vi "MPX Panel.vi"(8 "error in":errorcluster, 11 "session in":T1={"niScope"={"channel cfg"=[], "sessions"=[], "multi cards"=FALSE, "channels"=0, "type"=enum."n/a", "memory [B/chn]"=0, "ext. clock [Hz]"=0.0, "samples count"=0, "use streaming"=FALSE, "proc setup"={"packet size [smpl]"=0, "current timeout [s]"=0.0, "blk2blk timeout [s]"=0.0, "event time"=timestamp(0 s since 1904-01-01), "temp sampl T [s]"=0.0, "data queue"=refnum, "stop notifier"=refnum, "proc ref"=refnum}, "sample width [B]"=0, "ranges [V]"=[], "trigger setup"={"coupling"=1, "level [V]"=0.0, "slope"=0, "mode"=enum."Immediate"}, "fs [Hz]"=0.0, "bitres [bit]"=0, "clock source"=enum."VAL_NO_SOURCE"}, "3458A"={"channels"=[], "sync unit"={"VISA"="", "type"=enum."Picotest U6200A"}, "awg unit"={"type"=enum."Agilent 331xxA to 332xxA", "VISA"="", "enable 10MHz ref"=FALSE, "cmi ckd2"={"VISA"="", "clock source"=enum."Auto", "manual ref clk"=FALSE, "ref clock [Hz]"=0.0, "div mode"=enum."Set divisor directly"}, "cmi sync v3"={"VISA"="", "baud rate [bd/s]"=115200, "source"=enum."Auto", "hv range"=enum."1kV", "fsrc is fixed"=FALSE, "fsrc [Hz]"=10000000.0, "freq integ [s]"=1.0, "freq filter"=5, "trig level"=enum."TTL 5V", "chn1 mode"=enum."Source divider", "chn1 level"=enum."Positive 5V", "chn2 mode"=enum."Source divider", "chn2 level"=enum."Positive 5V", "chn2 div"=1, "chn3 mode"=enum."Chn 1 Active", "chn3 level"=enum."Positive 5V", "chn1 div entry"=enum."Calculate nearest divisor from measured fx", "chn1 dev limit [%]"=1.0, "chn1 check dev"=FALSE}, "trigger"={"source"=enum."Immediate", "level [V]"=0.0, "coupling"=enum."DC", "slope"=enum."POS"}, "HMF2500 cfg"={"Baud Rate"=9600, "Parity"=0, "Data Bits"=8, "Flow Control"=4}}, "sync mode"=enum."MASTER-SLAVE, MASTER clocked by TIMER", "streaming mode"=FALSE, "idn mode"=enum."Auto", "sampling mode"=enum."DCV", "sample memory [B]"=0, "proc setup"={"channel id"=0, "packet size [smpl]"=0, "current timeout [s]"=0.0, "blk2blk timeout [s]"=0.0, "event time"=timestamp(0 s since 1904-01-01), "stop notifier"=refnum, "data queues"=[], "proc refs"=[], "bus semaphore"=refnum}, "sample size [B]"=0, "sample count"=0, "aux data"={"channel id"=0, "valid?"=[], "gain [V]"=[], "timestamp [s]"=[], "Ts [s]"=0.0, "abs timestamp"=timestamp(0 s since 1904-01-01), "t [deg C]"=[], "multiplex timestamp [s]"=-1.0, "only multiplex?"=FALSE, "multiplex smpl offset"=0, "overflow?"=FALSE}, "ranges [V]"=[], "aperture [s]"=0.0, "LEVEL trigger"={"edge"=enum."POS", "level [V]"=0.0, "coupling"=enum."DC"}, "trigger mode"=enum."AUTO", "measure temp.?"=FALSE, "disp mesages"=[], "shared bus?"=FALSE, "disable display?"=FALSE, "aper mode"=enum."Manual", "aper rules"=[], "multiplex"={"cycles"=0, "delay [s]"=0.0, "enabled"=FALSE, "overhead [s]"=1.0, "tot smpls"=0, "sub-rec"=0, "overhead [%]"=0.0, "emulated"=FALSE}, "F8588 lpf"=enum."Off", "F8588 pll"=enum."Off", "F8588 couple"=enum."DC, auto", "fs"={"freq mode"=enum."fs or Ts", "fs [Hz]"=0.0, "fref [Hz]"=0.0, "mul"=0.0, "div"=0.0}}, "dsdll"={"dsdll"={"dsdll path"=path "", "dsdll handle"=[], "output devices"=[], "capture devices"=[]}, "channels"=0, "device id"=0, "channel idns"=[], "proc setup"={"packet size [smpl]"=0, "current timeout [s]"=0.0, "blk2blk timeout [s]"=0.0, "event time"=timestamp(0 s since 1904-01-01), "data queue"=refnum, "stop notifier"=refnum, "proc ref"=refnum}, "samples count"=0, "fs [Hz]"=0.0}, "type"=enum."niScope", "channel idn str"=[], "aux instr idn str"=[], "modified?"=FALSE, "simadc"={"channels"=[], "range [V]"=0.0, "Ts step [s]"=0.0, "time [s]"=0.0, "fs [Hz]"=0.0, "count"=0, "smpl offset"=0, "set count"=0, "bit res"=0}, "force rst?"=FALSE, "exit mode"=enum."Immediate reset", "exit dly"=0.0, "exit tmr"=timestamp(0 s since 1904-01-01), "busy?"=FALSE, "accessed?"=FALSE, "multiplex"={"Type"=enum."Dummy", "gen com ssn"={"visa"="", "primary"=enum."None", "secondary"=enum."None", "channels"=[]}, "delay before [s]"=0.0, "delay post [s]"=0.0, "sequence"=[], "enabled"=FALSE, "ref timestamp [s]"=0.0, "idn string"="", "dev niScope"="", "niScope idx"=0, "QPMX ssn"={"visa"="", "switch mode"=enum."Switched by TWM", "sequence"=[], "timing delays"=[], "polarity"=enum."Positive", "ss delay (s)"=2.0, "internal timer (s)"=1.0, "Last loaded sequence file"=path ""}, "VISA mux ssn"={"VISA"="", "paths"=[], "idn command"="", "serial cfg"={"Baud rate"=9600, "Data bits"=8, "Parity"=0, "Stop bits"=10, "Flow control"=0, "End Mode Read"=enum."None", "End Mode Write"=enum."None", "Term character"=0, "Term enable"=FALSE}}}, "keysight dso"={"VISA"="", "channels"=[], "bw limit [Hz]"=0.0, "resolution"=enum."Auto", "trig noise reject"=enum."Normal", "N"=0, "trigger config"={"trigger source"=enum."Immediate", "level [V]"=0.0, "trigger slope"=enum."Negative"}, "fs [Hz]"=0.0, "timeout stop"=timestamp(0 s since 1904-01-01), "waiting for opc"=FALSE, "fetch offset [smpl]"=0, "abs timestamp"=timestamp(0 s since 1904-01-01), "ranges [V]"=[]}, "cdaq"={"mclk [Hz]"=12800000.0, "ADC task"="", "mclk reference"="", "fs [Hz]"=50000.0, "queue adc cmd"=refnum, "queue adc data"=refnum, "adc proc ref"=refnum, "channels"=[], "last channels"=[], "timeout"=timestamp(0 s since 1904-01-01), "N"=1000, "mclk mode"=enum."Free running", "ext mclk source"=""}, "ignore overload"=FALSE} {"cdaq"."last channels"."Channel id" min=0 step=1; "cdaq"."channels"."Channel id" min=0 step=1; "keysight dso"."bw limit [Hz]" format="%#_6p"; "keysight dso"."channels"."Offset [V]" min=0.0 format="%#_6p"; "keysight dso"."channels"."Range [Vpk]" min=0.0 format="%#_6p"; "keysight dso"."channels"."Channel" min=1; "multiplex"."VISA mux ssn"."serial cfg"."Flow control" items=["None", "XON/XOFF", "CTS/RTS", "XON/XOFF + CTS/RTS", "DTR/DSR", "XON/XOFF + DTR/DSR"]; "multiplex"."VISA mux ssn"."serial cfg"."Stop bits" items=["1 bit"=10, "1.5 bits"=15, "2 bits"=20]; "multiplex"."VISA mux ssn"."serial cfg"."Parity" items=["None", "Odd", "Even", "Mark", "Space"]; "multiplex"."VISA mux ssn"."serial cfg"."Data bits" items=["5 bits"=5, "6 bits"=6, "7 bits"=7, "8 bits"=8]; "multiplex"."VISA mux ssn"."serial cfg"."Baud rate" items=["150 Bd"=150, "300 Bd"=300, "600 Bd"=600, "1200 Bd"=1200, "2400 Bd"=2400, "4800 Bd"=4800, "9600 Bd"=9600, "19.2 kBd"=19200, "38.4 kBd"=38400, "57.6 kBd"=57600, "115.2 kBd"=115200]; "multiplex"."QPMX ssn"."internal timer (s)" min=0.0 step=1.0; "multiplex"."QPMX ssn"."ss delay (s)" min=0.0 step=1.0; "multiplex"."QPMX ssn"."timing delays" min=1 max=255 step=1; "3458A"."awg unit"."HMF2500 cfg"."Flow Control" items=["None", "XON/XOFF", "RTS/CTS", "XON/XOFF & RTS/CTS", "DTR/DSR", "XON/XOFF & DTR/DSR"]; "3458A"."awg unit"."HMF2500 cfg"."Data Bits" items=["7"=7, "8"=8]; "3458A"."awg unit"."HMF2500 cfg"."Parity" items=["None", "Odd", "Even", "Mark", "Space"]; "3458A"."awg unit"."HMF2500 cfg"."Baud Rate" items=["300"=300, "600"=600, "1200"=1200, "2400"=2400, "4800"=4800, "9600"=9600, "19200"=19200]; "3458A"."awg unit"."cmi sync v3"."chn2 div" min=1 max=100000000 step=1; "3458A"."awg unit"."cmi sync v3"."fsrc [Hz]" format="%_8p"; "3458A"."channels"."Range [Vpk]" min=0.0; "niScope"."trigger setup"."level [V]" format="%.2f"; "niScope"."trigger setup"."coupling" items=["AC"=0, "DC"=1, "HF Reject"=3, "LF Reject"=4, "AC Plus HF Reject"=1001]; "niScope"."channel cfg"."Range [Vpk]" min=0.0; "niScope"."channel cfg"."Channel" min=0}) -> (0 "error out":errorcluster, 3 "session out":T1={"niScope"={"channel cfg"=[], "sessions"=[], "multi cards"=FALSE, "channels"=0, "type"=enum."n/a", "memory [B/chn]"=0, "ext. clock [Hz]"=0.0, "samples count"=0, "use streaming"=FALSE, "proc setup"={"packet size [smpl]"=0, "current timeout [s]"=0.0, "blk2blk timeout [s]"=0.0, "event time"=timestamp(0 s since 1904-01-01), "temp sampl T [s]"=0.0, "data queue"=refnum, "stop notifier"=refnum, "proc ref"=refnum}, "sample width [B]"=0, "ranges [V]"=[], "trigger setup"={"coupling"=1, "level [V]"=0.0, "slope"=0, "mode"=enum."Immediate"}, "fs [Hz]"=0.0, "bitres [bit]"=0, "clock source"=enum."VAL_NO_SOURCE"}, "3458A"={"channels"=[], "sync unit"={"VISA"="", "type"=enum."Picotest U6200A"}, "awg unit"={"type"=enum."Agilent 331xxA to 332xxA", "VISA"="", "enable 10MHz ref"=FALSE, "cmi ckd2"={"VISA"="", "clock source"=enum."Auto", "manual ref clk"=FALSE, "ref clock [Hz]"=0.0, "div mode"=enum."Set divisor directly"}, "cmi sync v3"={"VISA"="", "baud rate [bd/s]"=115200, "source"=enum."Auto", "hv range"=enum."1kV", "fsrc is fixed"=FALSE, "fsrc [Hz]"=10000000.0, "freq integ [s]"=1.0, "freq filter"=5, "trig level"=enum."TTL 5V", "chn1 mode"=enum."Source divider", "chn1 level"=enum."Positive 5V", "chn2 mode"=enum."Source divider", "chn2 level"=enum."Positive 5V", "chn2 div"=1, "chn3 mode"=enum."Chn 1 Active", "chn3 level"=enum."Positive 5V", "chn1 div entry"=enum."Calculate nearest divisor from measured fx", "chn1 dev limit [%]"=1.0, "chn1 check dev"=FALSE}, "trigger"={"source"=enum."Immediate", "level [V]"=0.0, "coupling"=enum."DC", "slope"=enum."POS"}, "HMF2500 cfg"={"Baud Rate"=9600, "Parity"=0, "Data Bits"=8, "Flow Control"=4}}, "sync mode"=enum."MASTER-SLAVE, MASTER clocked by TIMER", "streaming mode"=FALSE, "idn mode"=enum."Auto", "sampling mode"=enum."DCV", "sample memory [B]"=0, "proc setup"={"channel id"=0, "packet size [smpl]"=0, "current timeout [s]"=0.0, "blk2blk timeout [s]"=0.0, "event time"=timestamp(0 s since 1904-01-01), "stop notifier"=refnum, "data queues"=[], "proc refs"=[], "bus semaphore"=refnum}, "sample size [B]"=0, "sample count"=0, "aux data"={"channel id"=0, "valid?"=[], "gain [V]"=[], "timestamp [s]"=[], "Ts [s]"=0.0, "abs timestamp"=timestamp(0 s since 1904-01-01), "t [deg C]"=[], "multiplex timestamp [s]"=-1.0, "only multiplex?"=FALSE, "multiplex smpl offset"=0, "overflow?"=FALSE}, "ranges [V]"=[], "aperture [s]"=0.0, "LEVEL trigger"={"edge"=enum."POS", "level [V]"=0.0, "coupling"=enum."DC"}, "trigger mode"=enum."AUTO", "measure temp.?"=FALSE, "disp mesages"=[], "shared bus?"=FALSE, "disable display?"=FALSE, "aper mode"=enum."Manual", "aper rules"=[], "multiplex"={"cycles"=0, "delay [s]"=0.0, "enabled"=FALSE, "overhead [s]"=1.0, "tot smpls"=0, "sub-rec"=0, "overhead [%]"=0.0, "emulated"=FALSE}, "F8588 lpf"=enum."Off", "F8588 pll"=enum."Off", "F8588 couple"=enum."DC, auto", "fs"={"freq mode"=enum."fs or Ts", "fs [Hz]"=0.0, "fref [Hz]"=0.0, "mul"=0.0, "div"=0.0}}, "dsdll"={"dsdll"={"dsdll path"=path "", "dsdll handle"=[], "output devices"=[], "capture devices"=[]}, "channels"=0, "device id"=0, "channel idns"=[], "proc setup"={"packet size [smpl]"=0, "current timeout [s]"=0.0, "blk2blk timeout [s]"=0.0, "event time"=timestamp(0 s since 1904-01-01), "data queue"=refnum, "stop notifier"=refnum, "proc ref"=refnum}, "samples count"=0, "fs [Hz]"=0.0}, "type"=enum."niScope", "channel idn str"=[], "aux instr idn str"=[], "modified?"=FALSE, "simadc"={"channels"=[], "range [V]"=0.0, "Ts step [s]"=0.0, "time [s]"=0.0, "fs [Hz]"=0.0, "count"=0, "smpl offset"=0, "set count"=0, "bit res"=0}, "force rst?"=FALSE, "exit mode"=enum."Immediate reset", "exit dly"=0.0, "exit tmr"=timestamp(0 s since 1904-01-01), "busy?"=FALSE, "accessed?"=FALSE, "multiplex"={"Type"=enum."Dummy", "gen com ssn"={"visa"="", "primary"=enum."None", "secondary"=enum."None", "channels"=[]}, "delay before [s]"=0.0, "delay post [s]"=0.0, "sequence"=[], "enabled"=FALSE, "ref timestamp [s]"=0.0, "idn string"="", "dev niScope"="", "niScope idx"=0, "QPMX ssn"={"visa"="", "switch mode"=enum."Switched by TWM", "sequence"=[], "timing delays"=[], "polarity"=enum."Positive", "ss delay (s)"=2.0, "internal timer (s)"=1.0, "Last loaded sequence file"=path ""}, "VISA mux ssn"={"VISA"="", "paths"=[], "idn command"="", "serial cfg"={"Baud rate"=9600, "Data bits"=8, "Parity"=0, "Stop bits"=10, "Flow control"=0, "End Mode Read"=enum."None", "End Mode Write"=enum."None", "Term character"=0, "Term enable"=FALSE}}}, "keysight dso"={"VISA"="", "channels"=[], "bw limit [Hz]"=0.0, "resolution"=enum."Auto", "trig noise reject"=enum."Normal", "N"=0, "trigger config"={"trigger source"=enum."Immediate", "level [V]"=0.0, "trigger slope"=enum."Negative"}, "fs [Hz]"=0.0, "timeout stop"=timestamp(0 s since 1904-01-01), "waiting for opc"=FALSE, "fetch offset [smpl]"=0, "abs timestamp"=timestamp(0 s since 1904-01-01), "ranges [V]"=[]}, "cdaq"={"mclk [Hz]"=12800000.0, "ADC task"="", "mclk reference"="", "fs [Hz]"=50000.0, "queue adc cmd"=refnum, "queue adc data"=refnum, "adc proc ref"=refnum, "channels"=[], "last channels"=[], "timeout"=timestamp(0 s since 1904-01-01), "N"=1000, "mclk mode"=enum."Free running", "ext mclk source"=""}, "ignore overload"=FALSE} {"cdaq"."last channels"."Channel id" min=0 step=1; "cdaq"."channels"."Channel id" min=0 step=1; "keysight dso"."bw limit [Hz]" format="%#_6p"; "keysight dso"."channels"."Offset [V]" min=0.0 format="%#_6p"; "keysight dso"."channels"."Range [Vpk]" min=0.0 format="%#_6p"; "keysight dso"."channels"."Channel" min=1; "multiplex"."VISA mux ssn"."serial cfg"."Flow control" items=["None", "XON/XOFF", "CTS/RTS", "XON/XOFF + CTS/RTS", "DTR/DSR", "XON/XOFF + DTR/DSR"]; "multiplex"."VISA mux ssn"."serial cfg"."Stop bits" items=["1 bit"=10, "1.5 bits"=15, "2 bits"=20]; "multiplex"."VISA mux ssn"."serial cfg"."Parity" items=["None", "Odd", "Even", "Mark", "Space"]; "multiplex"."VISA mux ssn"."serial cfg"."Data bits" items=["5 bits"=5, "6 bits"=6, "7 bits"=7, "8 bits"=8]; "multiplex"."VISA mux ssn"."serial cfg"."Baud rate" items=["150 Bd"=150, "300 Bd"=300, "600 Bd"=600, "1200 Bd"=1200, "2400 Bd"=2400, "4800 Bd"=4800, "9600 Bd"=9600, "19.2 kBd"=19200, "38.4 kBd"=38400, "57.6 kBd"=57600, "115.2 kBd"=115200]; "multiplex"."QPMX ssn"."internal timer (s)" min=0.0 step=1.0; "multiplex"."QPMX ssn"."ss delay (s)" min=0.0 step=1.0; "multiplex"."QPMX ssn"."timing delays" min=1 max=255 step=1; "3458A"."awg unit"."HMF2500 cfg"."Flow Control" items=["None", "XON/XOFF", "RTS/CTS", "XON/XOFF & RTS/CTS", "DTR/DSR", "XON/XOFF & DTR/DSR"]; "3458A"."awg unit"."HMF2500 cfg"."Data Bits" items=["7"=7, "8"=8]; "3458A"."awg unit"."HMF2500 cfg"."Parity" items=["None", "Odd", "Even", "Mark", "Space"]; "3458A"."awg unit"."HMF2500 cfg"."Baud Rate" items=["300"=300, "600"=600, "1200"=1200, "2400"=2400, "4800"=4800, "9600"=9600, "19200"=19200]; "3458A"."awg unit"."cmi sync v3"."chn2 div" min=1 max=100000000 step=1; "3458A"."awg unit"."cmi sync v3"."fsrc [Hz]" format="%_8p"; "3458A"."channels"."Range [Vpk]" min=0.0; "niScope"."trigger setup"."level [V]" format="%.2f"; "niScope"."trigger setup"."coupling" items=["AC"=0, "DC"=1, "HF Reject"=3, "LF Reject"=4, "AC Plus HF Reject"=1001]; "niScope"."channel cfg"."Range [Vpk]" min=0.0; "niScope"."channel cfg"."Channel" min=0})   [LabVIEW 2020]
doc: "Multiplexer configuration panel."
uses:
  drivers/Multiplexers/Generic VISA commands/GVISA Mux Path Entry.ctl
  MPX Type.ctl
  drivers/Multiplexers/Generic COM/GCOMM Signal.ctl
  drivers/Multiplexers/Generic COM/GCOMM Virtual Channel.ctl
  drivers/Multiplexers/Generic COM/GCOMM Logic State.ctl
  ADC Session.ctl
  drivers/niScope/niScope Session.ctl
  drivers/niScope/niScope Virtual Channel Config.ctl
  drivers/niScope/niScope Virtual Channel Mode.ctl
  drivers/niScope/niScope Virtual Channel Input Z.ctl
  drivers/niScope/niScope Virtual Channel Coupling.ctl
  drivers/niScope/niScope Type.ctl
  drivers/niScope/niScope Digitizing Process Options.ctl
  drivers/niScope/niScope Data Packet.ctl
  drivers/niScope/niScope Trigger Setup.ctl
  <instrlib>/niScope/Controls/niScope trigger coupling.ctl
  <instrlib>/niScope/Controls/niScope trigger slope.ctl
  drivers/niScope/niScope Reference Clock.ctl
  drivers/DMM/3458A Digitizer Session.ctl
  drivers/DMM/3458A Virtual Channel Config.ctl
  drivers/Counter/Counter Session.ctl
  drivers/Counter/Counter Type.ctl
  drivers/AWG/AWG Session.ctl
  drivers/AWG/AWG Type.ctl
  drivers/AWG/CMI Clock Divider v2/CMI ckd2 Session.ctl
  drivers/AWG/CMI Clock Divider v2/CMI ckd2 Source Mode.ctl
  drivers/AWG/CMI Clock Divider v2/CMI ckd2 Divisor Mode.ctl
  drivers/AWG/CMI Sync V3/CMI Sync V3 session.ctl
  drivers/AWG/CMI Sync V3/Configure/CMI Sync V3 Reference Clock Source.ctl
  drivers/AWG/CMI Sync V3/Configure/CMI Sync V3 HV input Range.ctl
  drivers/AWG/CMI Sync V3/Configure/CMI Sync V3 Trigger Input Level.ctl
  drivers/AWG/CMI Sync V3/Configure/CMI Sync V3 Channel 1 Mode.ctl
  drivers/AWG/CMI Sync V3/Configure/CMI Sync V3 Channel Output Levels.ctl
  drivers/AWG/CMI Sync V3/Configure/CMI Sync V3 Channel 2 Mode.ctl
  drivers/AWG/CMI Sync V3/Configure/CMI Sync V3 Channel 3 Mode.ctl
  drivers/AWG/CMI Sync V3/Configure/CMI Sync V3 Channel 1 Divisor Entry Mode.ctl
  ADC Trig Config.ctl
  ADC Trig Mode Source.ctl
  ADC Trig Coupling.ctl
  ADC Trig Slope.ctl
  drivers/AWG/RaS HMF2500/HMF2500 Config.ctl
  drivers/DMM/3458A Sync Mode.ctl
  drivers/DMM/3458A Idn Mode.ctl
  drivers/DMM/3458A Digitizing Low Levels/Configure/Sampling Mode.ctl
  drivers/DMM/3458A Digitizing Process Options.ctl
  drivers/DMM/3458A Data Packet.ctl
  drivers/DMM/3458A Aux Record Data.ctl
  drivers/DMM/3458A Digitizing Low Levels/Configure/Level Setup.ctl
  drivers/DMM/3458A Digitizing Low Levels/Configure/First Sample Trigger.ctl
  drivers/DMM/3458A Aperture Selection Mode.ctl
  drivers/DMM/3458A Multiplexing Config.ctl
  drivers/Fluke 8588A/F8588A Low Pass Filter.ctl
  drivers/Fluke 8588A/F8588A Phase Lock.ctl
  drivers/Fluke 8588A/F8588A Coupling.ctl
  drivers/DMM/3458A Sampling Rate.ctl
  drivers/AWG/AWG Clock Setup Mode.ctl
  drivers/dsdll/DSDLL Session.ctl
  drivers/dsdll/dsdll/dsdll_instance.ctl
  drivers/dsdll/dsdll/dsdll_device_record.ctl
  drivers/dsdll/DSDLL Process Config.ctl
  drivers/dsdll/DSDLL Data Packet.ctl
  ADC Type.ctl
  drivers/simulated_adc/SimAdc Config.ctl
  drivers/simulated_adc/SimAdc Channel Cfg.ctl
  ADC On Close Action.ctl
  MPX Session.ctl
  drivers/Multiplexers/Generic COM/GCOMM Session.ctl
  drivers/Multiplexers/Generic COM/QPMX Session.ctl
  drivers/Multiplexers/QPMX/QPMX switch mode.ctl
  drivers/Multiplexers/QPMX/QPMX polarity.ctl
  drivers/Multiplexers/Generic VISA commands/GVISA Mux Session.ctl
  drivers/Multiplexers/Generic VISA commands/met_serial_setup.ctl
  drivers/Agilent DSO 90000/Virtual Digitizer/KeDSO session.ctl
  drivers/Agilent DSO 90000/Virtual Digitizer/KeDSO Virtual Channel.ctl
  drivers/Agilent DSO 90000/Virtual Digitizer/KeDSO Trigger Setup.ctl
  drivers/Agilent DSO 90000/Virtual Digitizer/KeDSO Trigger Source.ctl
  drivers/cdaq/cDAQ Session.ctl
  drivers/cdaq/low_level_old/cdaq_anal_adc_command.ctl
  drivers/cdaq/low_level_old/cdaq_anal_adc_data.ctl
  drivers/cdaq/cDAQ Virtual Channel.ctl
  drivers/cdaq/cDAQ Master Clock Mode.ctl
  varilib/SGUI Assign References Mode.ctl
  varilib/SGUI Assign Multiple Strings With Tags By Label.vi
  varilib/varilib.lvlib
  drivers/Multiplexers/QPMX/QuPMXLabVIEWdriver/QuPMXdriver.lvlib
  drivers/niScope/niScope Virtual Digitizer.lvlib
  drivers/DMM/3458A Virtual Digitizer.lvlib
  drivers/Counter/Counter.lvlib
  drivers/AWG/AWG.lvlib
  drivers/DMM/3458A Digitizing Low Levels/3458A Digitizing Low Levels.lvlib
  drivers/dsdll/DSDLL Virtual Digitizer.lvlib
  drivers/dsdll/dsdll/dsdll.lvlib
  drivers/AWG/CMI Sync V3/CMI Sync Unit V3.lvlib
panel:
  in  "tc device 2":enum32{"tc"}(tab) caption="Device"
  in  "btn set path":bool
  in  "man path":u16(ring) caption="Manual path select" items=["1"]
  in  "delay post":dbl caption="Delay after switch [s]" format="%#_3p"
  in  "delay pre":dbl caption="Delay before switch [s]" format="%#_3p"
  in  "sequence":T78(array[cluster]) caption="Sequence definition" {"Channel" items=["1"]}
  in  "btn idn":bool
  out "mpxstr":string caption="Identification/Status:"
  in  "btn cancel":bool
  in  "btn ok":bool
  in  "tc device":T79(tab) caption="Device"
  in  "com sec":T62 caption="Secondary signal"
  in  "com prim":T62 caption="Primary signal"
  in  "gen com visa":refnum<visa-resource-name> caption="Device VISA"
  in  "com chan":T63[](array[typedef]) caption="Virtual channel definitions"
  in  "niScope vchn":i32=1 caption="Index of niScope digitizer virtual channel whose PFI will be controlled" min=0
  in  "btn gen visa cfg com":bool
  in  "gen visa idn cmd":string caption="Identification command (optional, leave empty if not supported)"
  in  "gen visa visa":refnum<visa-resource-name> caption="Device VISA"
  in  "gen visa chans":T69[](array[typedef]) caption="Virtual channel definitions"
  out "qpmx loaded sequences":u32 caption="Sequences actually loaded in TWM:"
  in  "qpmx int timer":i32=1000 caption="Internal timer [ms]" min=0 step=1
  in  "qpmx load":bool caption="Load"
  in  "qpmx visa":refnum<visa-resource-name> caption="Multiplexer VISA"
  in  "qpmx file":path=path "D:/martin/QPsw - github/QuPMX/seqtest" caption="Sequence file path."
  in  "qpmx mode":T66 caption="Switch mode"
  in  "qpmx ss delay":dbl=20.0 caption="Short circuit delay [ms]" min=0.0 step=1.0
  in  "qpmx polarity":T67 caption="Triger polarity"
  in  "Type":T60
  # "Simple multiplexer control via PFI lines of 5922 (or similar). 5922 cannot directly set logic level to PFIs, but it can export reference clock (10 MHz) to it. The control logic signal level can be extracted by rectifying the clock by schottky diode and small capacitor. Rectified voltage logic levels will be 0 and roughly 3V.\n\nNote 1: The clock can be exported only if external reference clock is connected to 5922!\nNote 2: This multiplexer driver uses niScope digitizer virtual channels, so niScope must be selected as a digitizer and phase locked to external clock."
  # "Synchronous multiplexer from project Quantum Power with own clock or driven by external trigger signal.\nA multiplexing sequence have to be loaded into the multiplexer from a file."
  # "The Sequence definition is made automatically based on the loaded file.\nDO NOT change the Sequence definition!"
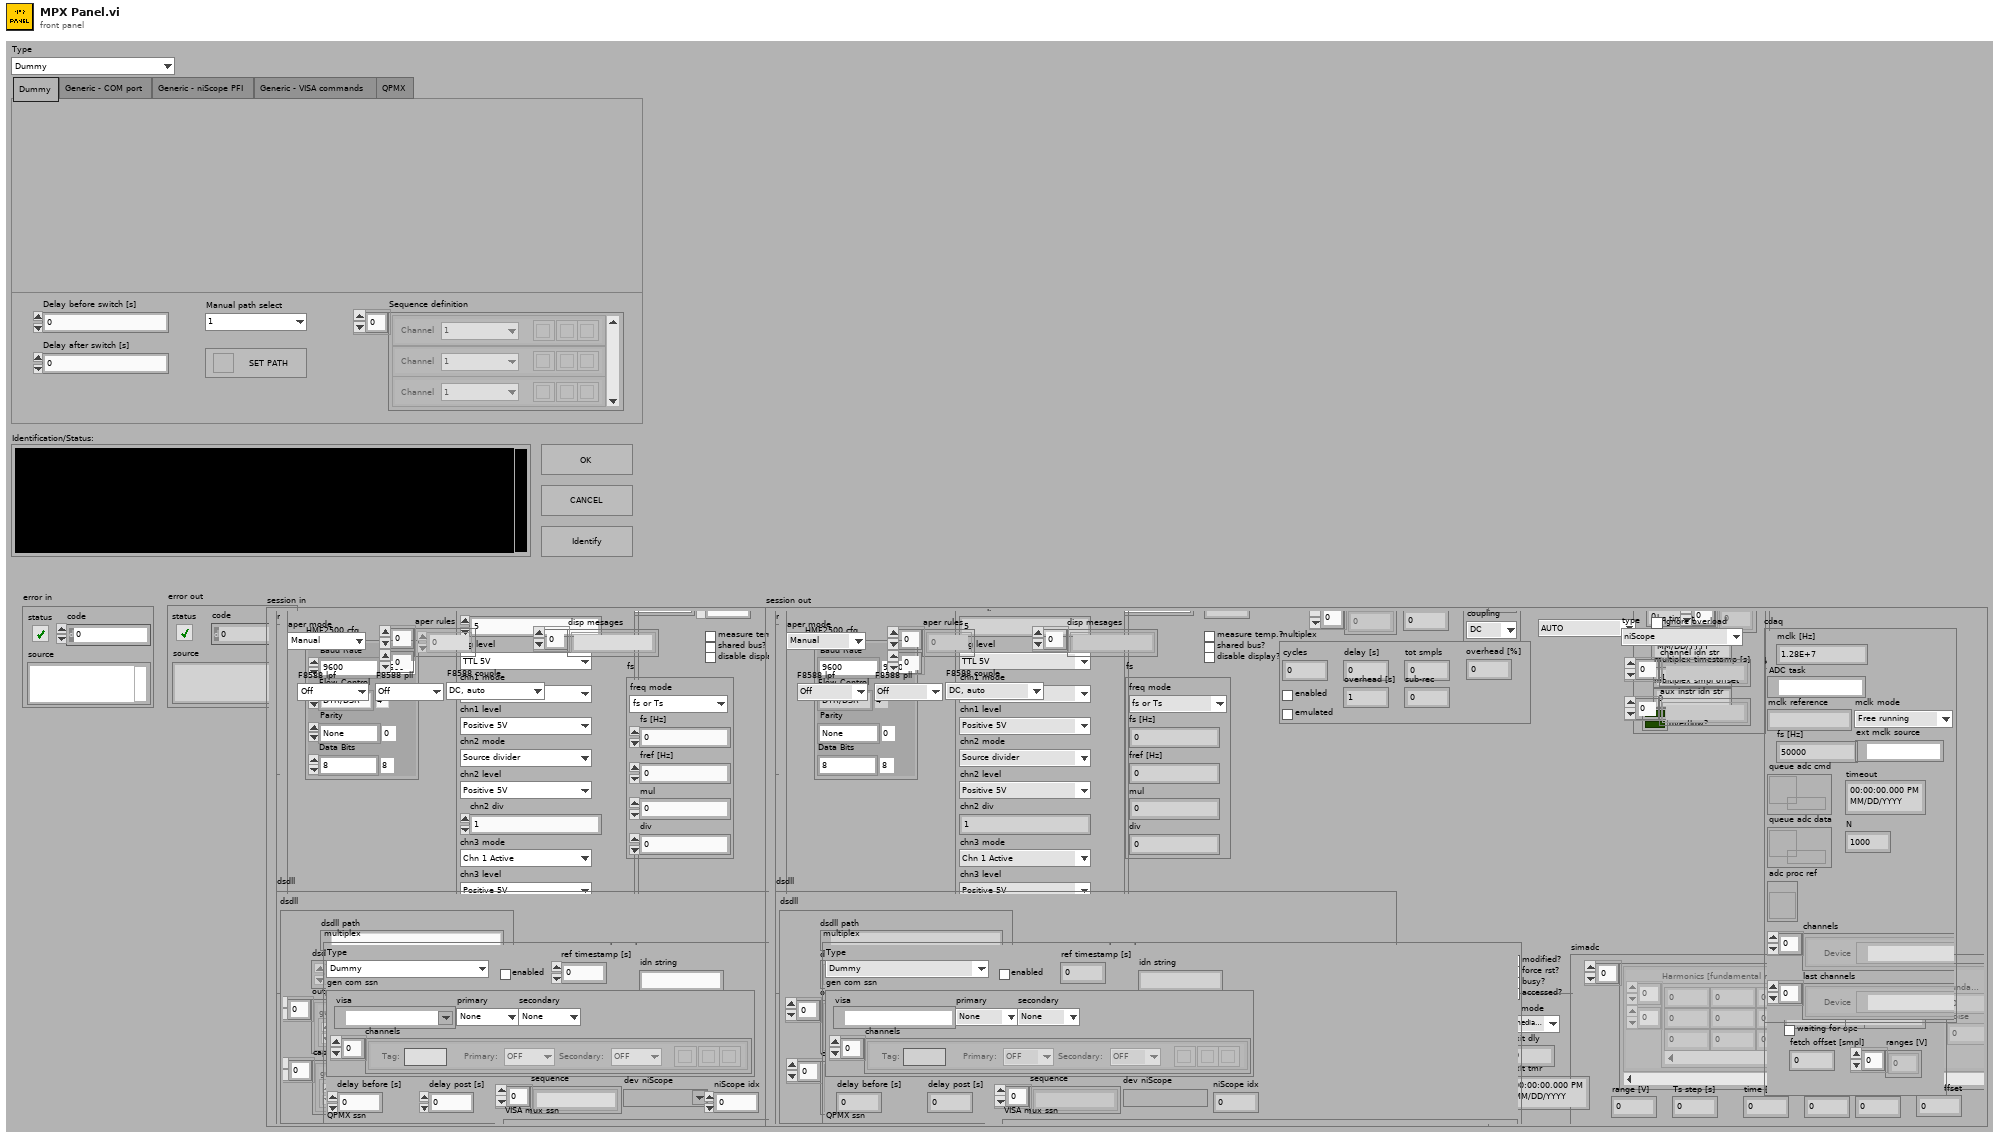
[diagram p1: front panel]
types:
  T1 = typedef "ADC Session.ctl" = cluster{"niScope":T2, "3458A":T13, "dsdll":T51, "type":T55, "channel idn str":string[], "aux instr idn str":string[], "modified?":bool, "simadc":T56, "force rst?":bool, "exit mode":T58, "exit dly":dbl, "exit tmr":timestamp, "busy?":bool, "accessed?":bool, "multiplex":T59, "keysight dso":T71, "cdaq":T75, "ignore overload":bool}
  T2 = typedef "niScope Virtual Digitizer.lvlib/niScope Session.ctl" = cluster{"channel cfg":T3[], "sessions":refnum<k20>[], "multi cards":bool, "channels":i32, "type":T7, "memory [B/chn]":i32, "ext. clock [Hz]":dbl, "samples count":i64, "use streaming":bool, "proc setup":T8, "sample width [B]":i32, "ranges [V]":dbl[], "trigger setup":T9, "fs [Hz]":dbl, "bitres [bit]":i32, "clock source":T12}
  T3 = typedef "niScope Virtual Digitizer.lvlib/niScope Virtual Channel Config.ctl" = cluster{"Address":refnum<k15>, "Channel":i32, "Mode":T4, "Input Z":T5, "Coupling":T6, "Range [Vpk]":dbl, "btn clr":bool, "btn up":bool, "btn down":bool}
  T4 = typedef "niScope Virtual Digitizer.lvlib/niScope Virtual Channel Mode.ctl" = enum16{"Single ended", "Unbal. differential", "Differential"}
  T5 = typedef "niScope Virtual Digitizer.lvlib/niScope Virtual Channel Input Z.ctl" = enum16{"1 MOhm", "50 Ohm"}
  T6 = typedef "niScope Virtual Digitizer.lvlib/niScope Virtual Channel Coupling.ctl" = enum16{"AC", "DC", "GND"}
  T7 = typedef "niScope Virtual Digitizer.lvlib/niScope Type.ctl" = enum16{"n/a", "5922"}
  T8 = typedef "niScope Virtual Digitizer.lvlib/niScope Digitizing Process Options.ctl" = cluster{"packet size [smpl]":i64, "current timeout [s]":dbl, "blk2blk timeout [s]":dbl, "event time":timestamp, "temp sampl T [s]":dbl, "data queue":refnum<queue>, "stop notifier":refnum<notifier>, "proc ref":refnum<vi>}
  T9 = typedef "niScope Virtual Digitizer.lvlib/niScope Trigger Setup.ctl" = cluster{"coupling":T10, "level [V]":dbl, "slope":T11, "mode":enum16{"Immediate", "External", "Level"}}
  T10 = typedef "niScope trigger coupling.ctl" = u16
  T11 = typedef "niScope trigger slope.ctl" = i32
  T12 = typedef "niScope Virtual Digitizer.lvlib/niScope Reference Clock.ctl" = enum16{"VAL_NO_SOURCE", "VAL_CLK_IN", "VAL_PXI_CLOCK", "VAL_EXTERNAL"}
  T13 = typedef "3458A Virtual Digitizer.lvlib/3458A Digitizer Session.ctl" = cluster{"channels":T14[], "sync unit":T15, "awg unit":T17, "sync mode":T36, "streaming mode":bool, "idn mode":T37, "sampling mode":T38, "sample memory [B]":i32, "proc setup":T39, "sample size [B]":i32, "sample count":i32, "aux data":T41, "ranges [V]":dbl[], "aperture [s]":dbl, "LEVEL trigger":T42, "trigger mode":T43, "measure temp.?":bool, "disp mesages":string[], "shared bus?":bool, "disable display?":bool, "aper mode":T44, "aper rules":dbl[][], "multiplex":T45, "F8588 lpf":T46, "F8588 pll":T47, "F8588 couple":T48, "fs":T49}
  T14 = typedef "3458A Virtual Digitizer.lvlib/3458A Virtual Channel Config.ctl" = cluster{"VISA":refnum<visa-resource-name>, "Range [Vpk]":dbl, "btn clr":bool, "btn up":bool, "btn down":bool, "F8588":bool, "F8588 guard":bool}
  T15 = typedef "Counter.lvlib/Counter Session.ctl" = cluster{"VISA":refnum<visa-resource-name>, "type":T16}
  T16 = typedef "Counter.lvlib/Counter Type.ctl" = enum16{"Picotest U6200A", "dummy"}
  T17 = typedef "AWG.lvlib/AWG Session.ctl" = cluster{"type":T18, "VISA":refnum<visa-resource-name>, "enable 10MHz ref":bool, "cmi ckd2":T19, "cmi sync v3":T22, "trigger":T31, "HMF2500 cfg":T35}
  T18 = typedef "AWG.lvlib/AWG Type.ctl" = enum16{"Agilent 331xxA to 332xxA", "Agilent 335xxA to 336xxA", "Tektronix AFG3101C", "R&S HMF25xx", "CMI Clock Divider v2", "CMI Sync Unit V3", "dummy"}
  T19 = typedef "AWG.lvlib/CMI ckd2 Session.ctl" = cluster{"VISA":refnum<visa-resource-name>, "clock source":T20, "manual ref clk":bool, "ref clock [Hz]":dbl, "div mode":T21}
  T20 = typedef "AWG.lvlib/CMI ckd2 Source Mode.ctl" = enum16{"Auto", "LF clock", "HF clock", "Internal"}
  T21 = typedef "AWG.lvlib/CMI ckd2 Divisor Mode.ctl" = enum16{"Set divisor directly", "Set divisor by frequency"}
  T22 = typedef "AWG.lvlib/CMI Sync Unit V3.lvlib/CMI Sync V3 session.ctl" = cluster{"VISA":refnum<visa-resource-name>, "baud rate [bd/s]":i32, "source":T23, "hv range":T24, "fsrc is fixed":bool, "fsrc [Hz]":dbl, "freq integ [s]":dbl, "freq filter":i32, "trig level":T25, "chn1 mode":T26, "chn1 level":T27, "chn2 mode":T28, "chn2 level":T27, "chn2 div":i32, "chn3 mode":T29, "chn3 level":T27, "chn1 div entry":T30, "chn1 dev limit [%]":dbl, "chn1 check dev":bool}
  T23 = typedef "AWG.lvlib/CMI Sync Unit V3.lvlib/CMI Sync V3 Reference Clock Source.ctl" = enum16{"Auto", "Internal", "Logic", "Sine", "HV"}
  T24 = typedef "AWG.lvlib/CMI Sync Unit V3.lvlib/CMI Sync V3 HV input Range.ctl" = enum16{"10V", "60V", "250V", "1kV"}
  T25 = typedef "AWG.lvlib/CMI Sync Unit V3.lvlib/CMI Sync V3 Trigger Input Level.ctl" = enum16{"LVCMOS 3V3", "TTL 5V"}
  T26 = typedef "AWG.lvlib/CMI Sync Unit V3.lvlib/CMI Sync V3 Channel 1 Mode.ctl" = enum16{"Source divider", "DDS absolute", "DDS ratio", "DDS ratio M/N"}
  T27 = typedef "AWG.lvlib/CMI Sync Unit V3.lvlib/CMI Sync V3 Channel Output Levels.ctl" = enum16{"Positive 3V3", "Negative 3V3", "Positive 5V", "Negative 5V"}
  T28 = typedef "AWG.lvlib/CMI Sync Unit V3.lvlib/CMI Sync V3 Channel 2 Mode.ctl" = enum16{"Source divider", "Chn 1 divide"}
  T29 = typedef "AWG.lvlib/CMI Sync Unit V3.lvlib/CMI Sync V3 Channel 3 Mode.ctl" = enum16{"Chn 1 Active", "Chn 2 Active", "Chn 1 Trigger", "Chn 2 Trigger", "Gate", "PPS", "10MHz"}
  T30 = typedef "AWG.lvlib/CMI Sync Unit V3.lvlib/CMI Sync V3 Channel 1 Divisor Entry Mode.ctl" = enum16{"Set divisor directly", "Calculate nearest divisor from measured fx"}
  T31 = typedef "ADC Trig Config.ctl" = cluster{"source":T32, "level [V]":dbl, "coupling":T33, "slope":T34}
  T32 = typedef "ADC Trig Mode Source.ctl" = enum16{"Immediate", "External", "Level"}
  T33 = typedef "ADC Trig Coupling.ctl" = enum16{"DC", "AC"}
  T34 = typedef "ADC Trig Slope.ctl" = enum16{"POS", "NEG"}
  T35 = typedef "AWG.lvlib/HMF2500 Config.ctl" = cluster{"Baud Rate":u32, "Parity":u16, "Data Bits":u16, "Flow Control":u16}
  T36 = typedef "3458A Virtual Digitizer.lvlib/3458A Sync Mode.ctl" = enum16{"MASTER-SLAVE, MASTER clocked by TIMER", "MASTER-SLAVE, MASTER clocked by AWG", "ALL clocked by AWG", "MASTER-SLAVE, ALL clocked by TIMER", "ALL clocked by AWG with DFLL"}
  T37 = typedef "3458A Virtual Digitizer.lvlib/3458A Idn Mode.ctl" = enum16{"Auto", "Sequential (chn A, chn B, ...)", "From calibration string"}
  T38 = typedef "3458A Virtual Digitizer.lvlib/3458A Digitizing Low Levels.lvlib/Sampling Mode.ctl" = enum16{"DCV", "DSDC", "DSAC"}
  T39 = typedef "3458A Virtual Digitizer.lvlib/3458A Digitizing Process Options.ctl" = cluster{"channel id":i32, "packet size [smpl]":i32, "current timeout [s]":dbl, "blk2blk timeout [s]":dbl, "event time":timestamp, "stop notifier":refnum<notifier>, "data queues":refnum<queue>[], "proc refs":refnum<vi>[], "bus semaphore":T40}
  T40 = typedef "Semaphore RefNum" = refnum<k1>
  T41 = typedef "3458A Virtual Digitizer.lvlib/3458A Aux Record Data.ctl" = cluster{"channel id":i32, "valid?":bool[], "gain [V]":dbl[], "timestamp [s]":dbl[], "Ts [s]":dbl, "abs timestamp":timestamp, "t [deg C]":dbl[], "multiplex timestamp [s]":dbl, "only multiplex?":bool, "multiplex smpl offset":i64, "overflow?":bool}
  T42 = typedef "3458A Virtual Digitizer.lvlib/3458A Digitizing Low Levels.lvlib/Level Setup.ctl" = cluster{"edge":enum16{"POS", "NEG"}, "level [V]":dbl, "coupling":enum16{"DC", "AC"}}
  T43 = typedef "3458A Virtual Digitizer.lvlib/3458A Digitizing Low Levels.lvlib/First Sample Trigger.ctl" = enum16{"AUTO", "EXT", "SYN", "SGL", "HOLD", "LEVEL"}
  T44 = typedef "3458A Virtual Digitizer.lvlib/3458A Aperture Selection Mode.ctl" = enum16{"Manual", "Maximum", "Table"}
  T45 = typedef "3458A Virtual Digitizer.lvlib/3458A Multiplexing Config.ctl" = cluster{"cycles":i32, "delay [s]":dbl, "enabled":bool, "overhead [s]":dbl, "tot smpls":i64, "sub-rec":i32, "overhead [%]":dbl, "emulated":bool}
  T46 = typedef "F8588A Low Pass Filter.ctl" = enum16{"Off", "100 kHz", "3 MHz"}
  T47 = typedef "F8588A Phase Lock.ctl" = enum16{"Off", "1 MHz", "10 MHz"}
  T48 = typedef "F8588A Coupling.ctl" = enum16{"AC, 1 MOhm", "AC, 10 MOhm", "DC, 1 MOhm", "DC, 10 MOhm", "DC, auto"}
  T49 = typedef "3458A Virtual Digitizer.lvlib/3458A Sampling Rate.ctl" = cluster{"freq mode":T50, "fs [Hz]":dbl, "fref [Hz]":dbl, "mul":dbl, "div":dbl}
  T50 = typedef "AWG.lvlib/AWG Clock Setup Mode.ctl" = enum16{"fs or Ts", "fs or Ts with fref", "fref/N", "fref*M/N", "fref*Ratio"}
  T51 = typedef "DSDLL Virtual Digitizer.lvlib/DSDLL Session.ctl" = cluster{"dsdll":T52, "channels":i32, "device id":i32, "channel idns":string[], "proc setup":T54, "samples count":i32, "fs [Hz]":dbl}
  T52 = typedef "dsdll.lvlib/dsdll_instance.ctl" = cluster{"dsdll path":path, "dsdll handle":u8[], "output devices":T53[], "capture devices":T53[]}
  T53 = typedef "dsdll.lvlib/dsdll_device_record.ctl" = cluster{"guid":u8[], "name":string}
  T54 = typedef "DSDLL Virtual Digitizer.lvlib/DSDLL Process Config.ctl" = cluster{"packet size [smpl]":i32, "current timeout [s]":dbl, "blk2blk timeout [s]":dbl, "event time":timestamp, "data queue":refnum<queue>, "stop notifier":refnum<notifier>, "proc ref":refnum<vi>}
  T55 = typedef "ADC Type.ctl" = enum16{"niScope", "3458A", "DirectSound DLL", "Keysight DSO", "cDAQ ADC", "dummy"}
  T56 = typedef "SimAdc Config.ctl" = cluster{"channels":T57[], "range [V]":dbl, "Ts step [s]":dbl, "time [s]":dbl, "fs [Hz]":dbl, "count":i64, "smpl offset":i64, "set count":i64, "bit res":i32}
  T57 = typedef "SimAdc Channel Cfg.ctl" = cluster{"harmonics":dbl[][], "btn clear":bool, "noise":dbl, "fundamental [Hz]":dbl}
  T58 = typedef "ADC On Close Action.ctl" = enum16{"Immediate reset", "Delayed reset"}
  T59 = typedef "MPX Session.ctl" = cluster{"Type":T60, "gen com ssn":T61, "delay before [s]":dbl, "delay post [s]":dbl, "sequence":string[], "enabled":bool, "ref timestamp [s]":dbl, "idn string":string, "dev niScope":refnum<k15>, "niScope idx":i32, "QPMX ssn":T65, "VISA mux ssn":T68}
  T60 = typedef "MPX Type.ctl" = enum16{"Dummy", "Generic - COM port", "Generic - niScope PFI", "Generic - VISA commands", "QPMX"}
  T61 = typedef "GCOMM Session.ctl" = cluster{"visa":refnum<visa-resource-name>, "primary":T62, "secondary":T62, "channels":T63[]}
  T62 = typedef "GCOMM Signal.ctl" = enum16{"None", "DTR", "RTS"}
  T63 = typedef "GCOMM Virtual Channel.ctl" = cluster{"Primary:":T64, "Secondary:":T64, "btn clr":bool, "btn up":bool, "btn down":bool, "Tag:":string}
  T64 = typedef "GCOMM Logic State.ctl" = enum16{"OFF", "ON"}
  T65 = typedef "QPMX Session.ctl" = cluster{"visa":refnum<visa-resource-name>, "switch mode":T66, "sequence":bool[][], "timing delays":u32[], "polarity":T67, "ss delay (s)":dbl, "internal timer (s)":dbl, "Last loaded sequence file":path}
  T66 = typedef "QPMX switch mode.ctl" = enum16{"Switched by TWM", "Switched by external clock", "Switched by internal clock"}
  T67 = typedef "QPMX polarity.ctl" = enum16{"Positive", "Negative"}
  T68 = typedef "GVISA Mux Session.ctl" = cluster{"VISA":refnum<visa-resource-name>, "paths":T69[], "idn command":string, "serial cfg":T70}
  T69 = typedef "GVISA Mux Path Entry.ctl" = cluster{"Tag:":string, "Command:":string, "btn clr":bool, "btn up":bool, "btn down":bool}
  T70 = typedef "met_serial_setup.ctl" = cluster{"Baud rate":i32, "Data bits":i32, "Parity":i32, "Stop bits":i32, "Flow control":i32, "End Mode Read":enum16{"None", "Last Bit", "TermChar"}, "End Mode Write":enum16{"None", "Last Bit", "TermChar"}, "Term character":u8, "Term enable":bool}
  T71 = typedef "KeDSO session.ctl" = cluster{"VISA":refnum<visa-resource-name>, "channels":T72[], "bw limit [Hz]":dbl, "resolution":enum16{"Auto", "Bits 9", "Bits 10", "Bits 11", "Bits 12"}, "trig noise reject":enum16{"Normal", "High Sensitivity"}, "N":i64, "trigger config":T73, "fs [Hz]":dbl, "timeout stop":timestamp, "waiting for opc":bool, "fetch offset [smpl]":i64, "abs timestamp":timestamp, "ranges [V]":dbl[]}
  T72 = typedef "KeDSO Virtual Channel.ctl" = cluster{"Channel":i32, "Range [Vpk]":dbl, "btn clr":bool, "btn up":bool, "btn down":bool, "Offset [V]":dbl, "Coupling":enum16{"DC", "DC50", "AC", "LFR1"}, "bw limit enab":bool}
  T73 = typedef "KeDSO Trigger Setup.ctl" = cluster{"trigger source":T74, "level [V]":dbl, "trigger slope":enum16{"Negative", "Positive", "Either"}}
  T74 = typedef "KeDSO Trigger Source.ctl" = enum16{"Immediate", "Level", "AUX"}
  T75 = typedef "cDAQ Session.ctl" = cluster{"mclk [Hz]":dbl, "ADC task":refnum<k21>, "mclk reference":string, "fs [Hz]":dbl, "queue adc cmd":refnum<queue>, "queue adc data":refnum<queue>, "adc proc ref":refnum<vi>, "channels":T76[], "last channels":T76[], "timeout":timestamp, "N":i32, "mclk mode":T77, "ext mclk source":tag}
  T76 = typedef "cDAQ Virtual Channel.ctl" = cluster{"Device":tag, "Channel id":i32, "btn clr":bool, "btn up":bool, "btn down":bool}
  T77 = typedef "cDAQ Master Clock Mode.ctl" = enum16{"Free running", "Export master clock", "Import master clock"}
  T78 = cluster{"btn clr":bool, "btn up":bool, "btn down":bool, "Channel":u16}[]
  T79 = enum32{"Dummy", "Generic - COM port", "Generic - niScope PFI", "Generic - VISA commands", "QPMX"}
  T80 = typedef "varilib.lvlib/SGUI Assign References Mode.ctl" = enum16{"Add to stack", "Overwrite", "Release last", "Release ID"}
  T81 = cluster{"btn clr":bool, "btn up":bool, "btn down":bool, "Channel":u16}
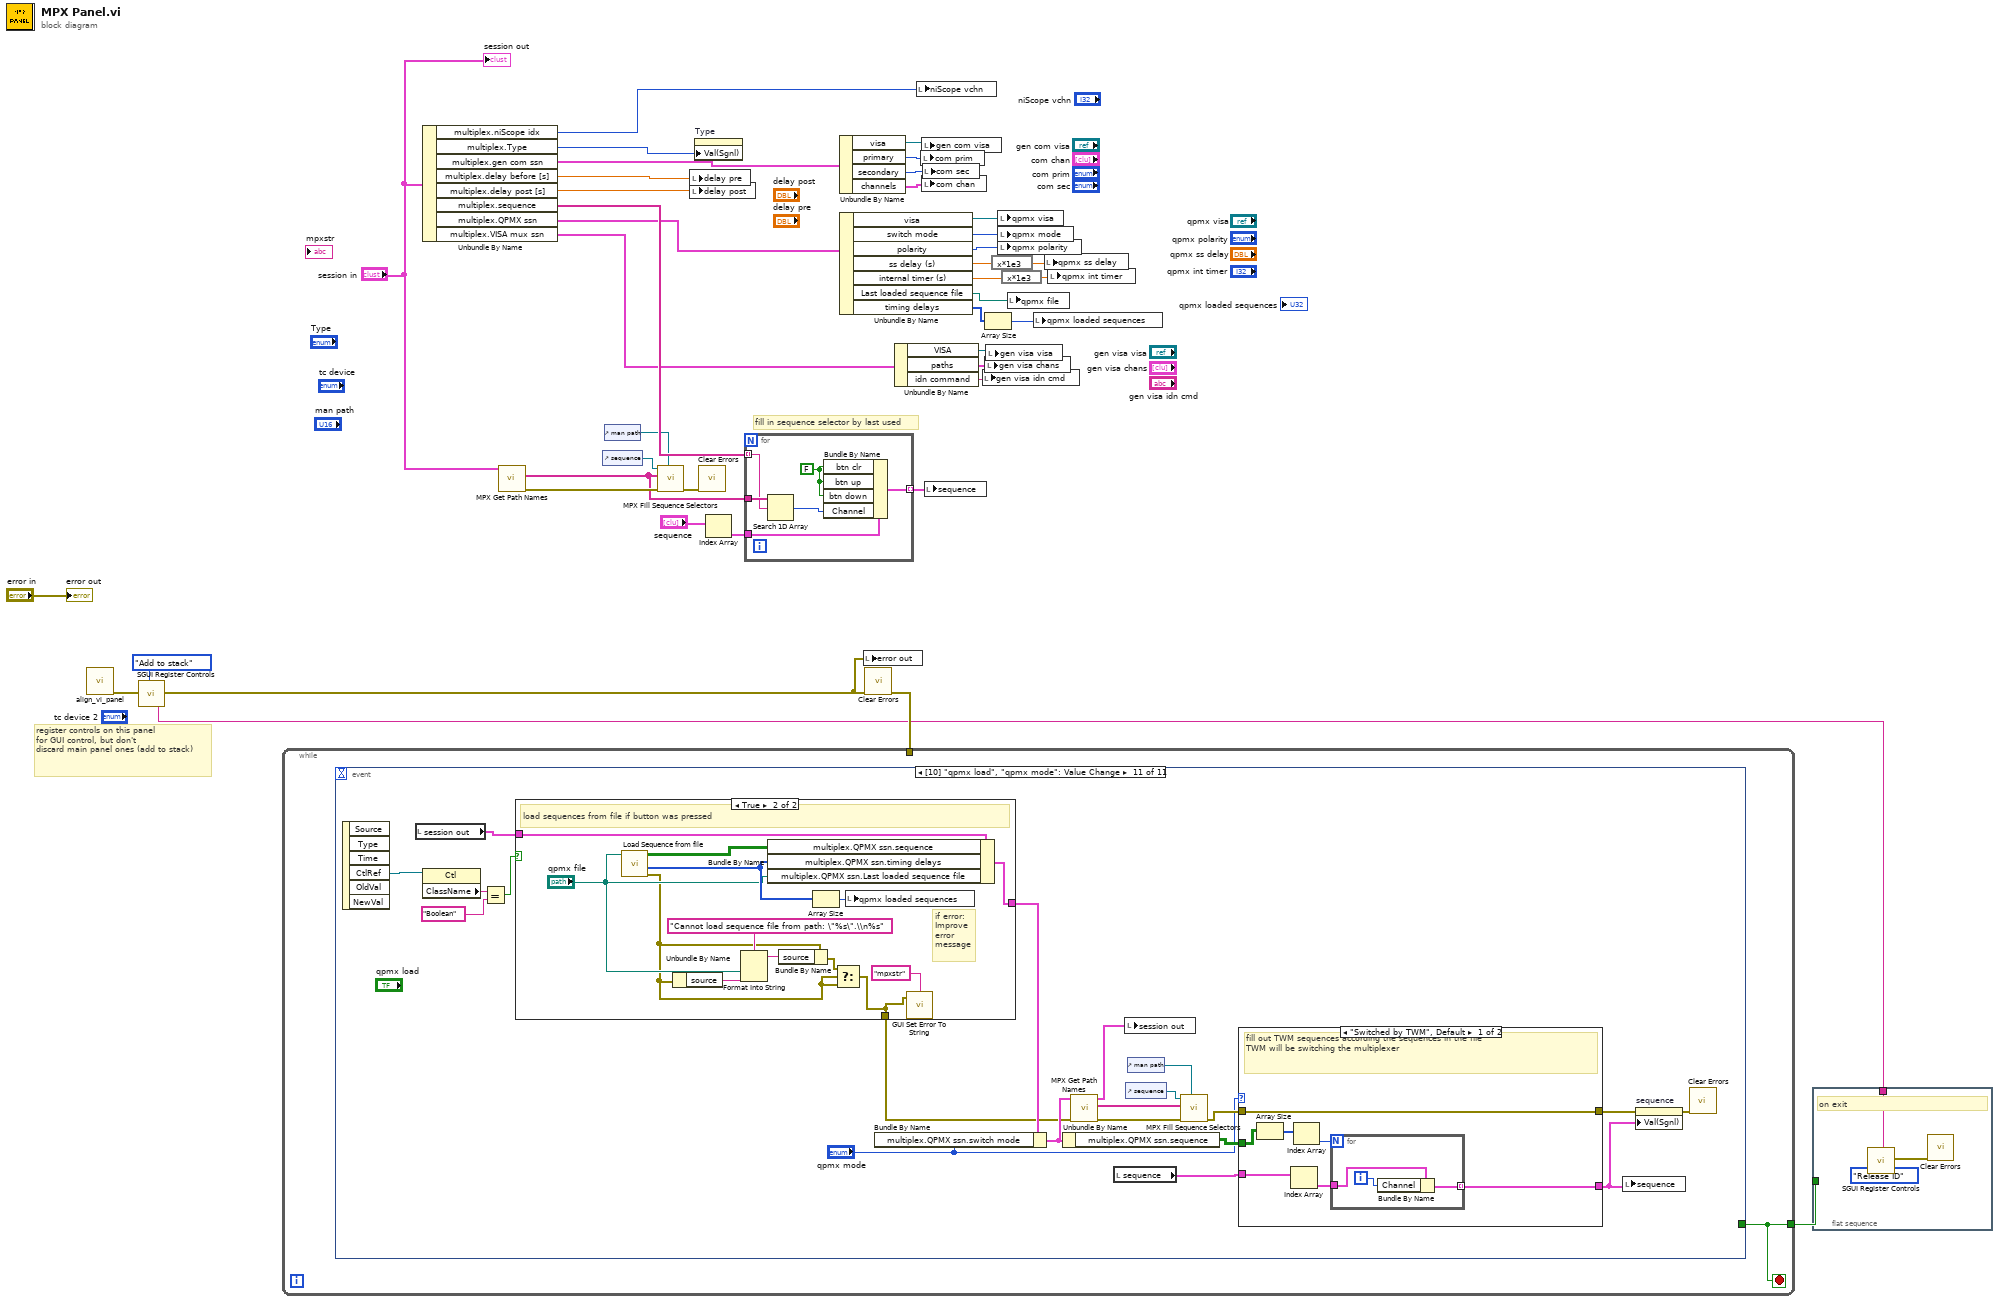
[diagram p0: block diagram]
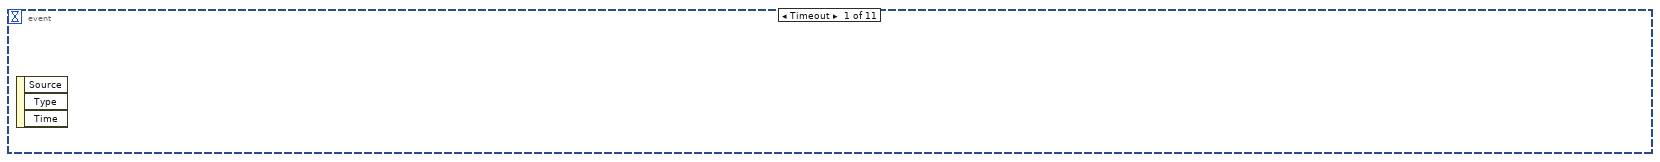
[diagram p2: hidden frame]
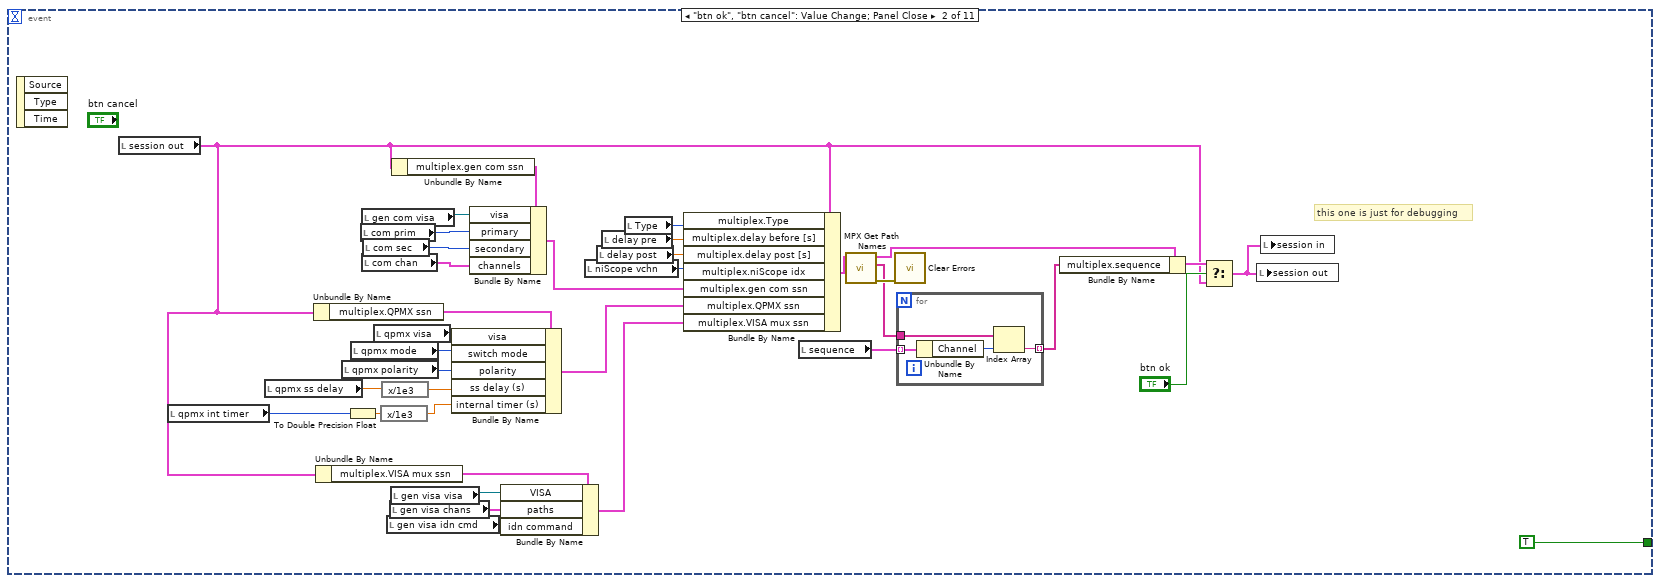
[diagram p3: hidden frame]
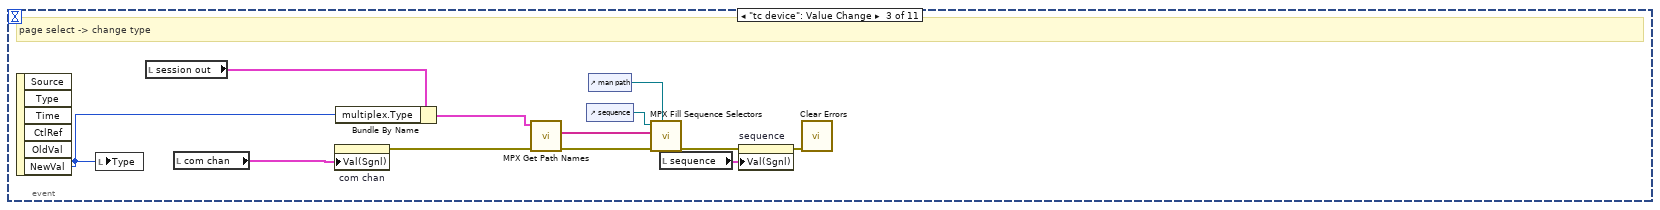
[diagram p4: hidden frame]
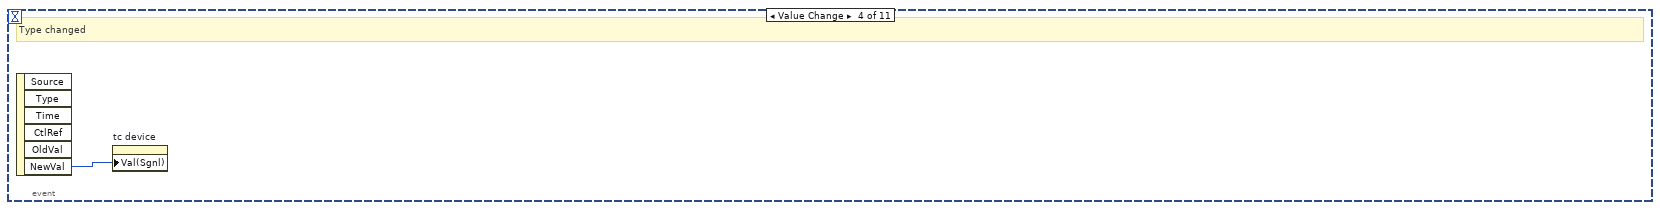
[diagram p5: hidden frame]
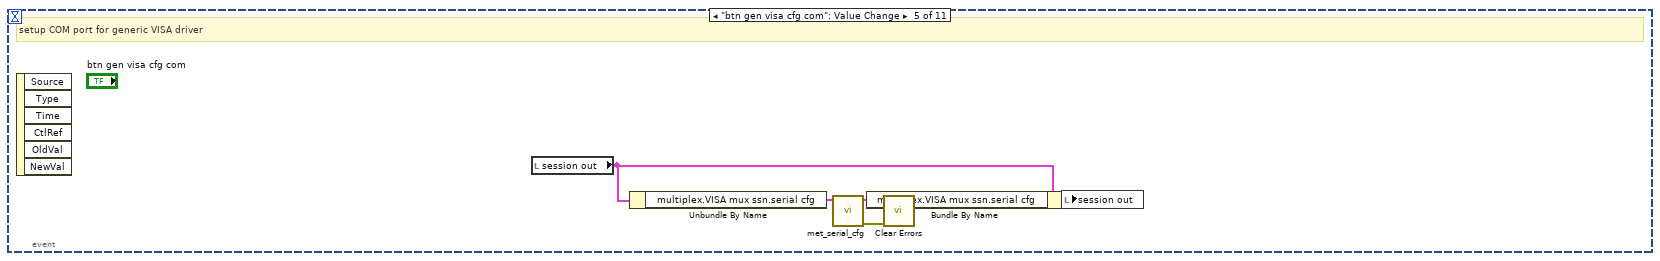
[diagram p6: hidden frame]
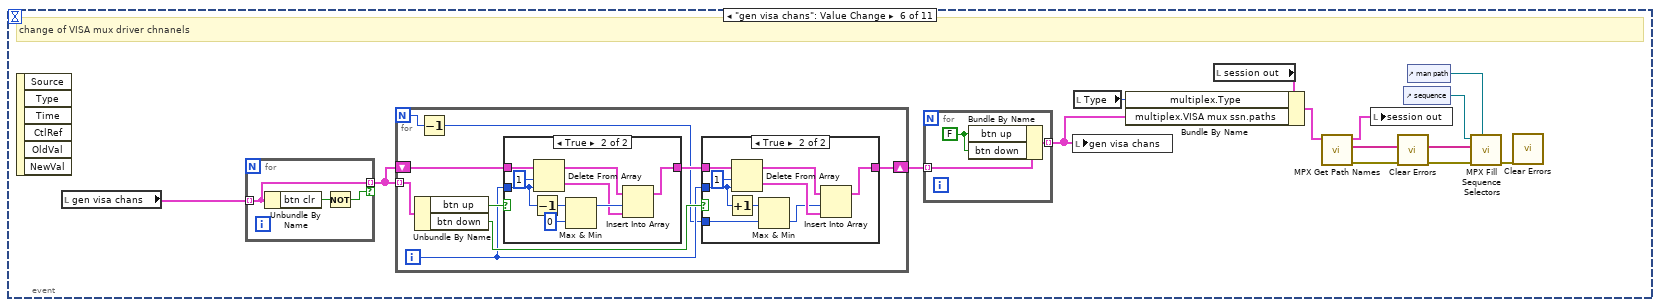
[diagram p7: hidden frame]
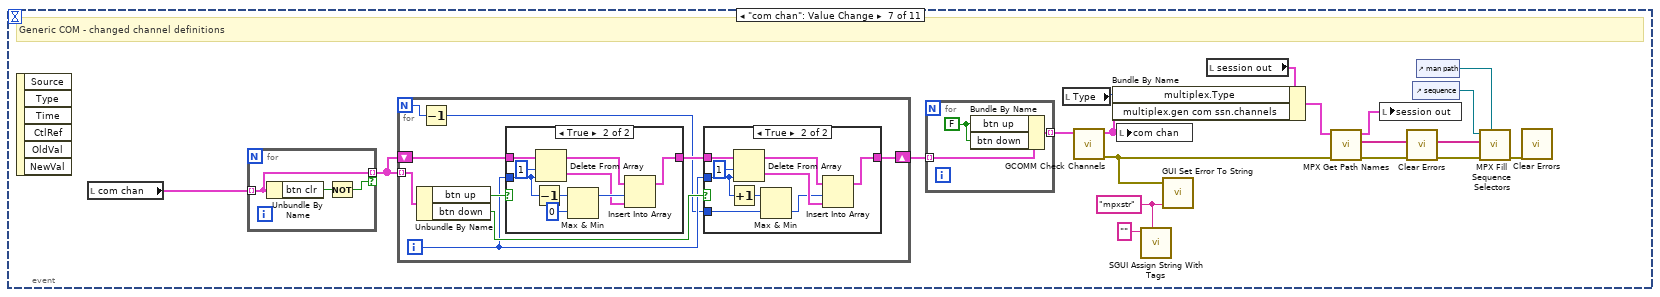
[diagram p10: hidden frame]
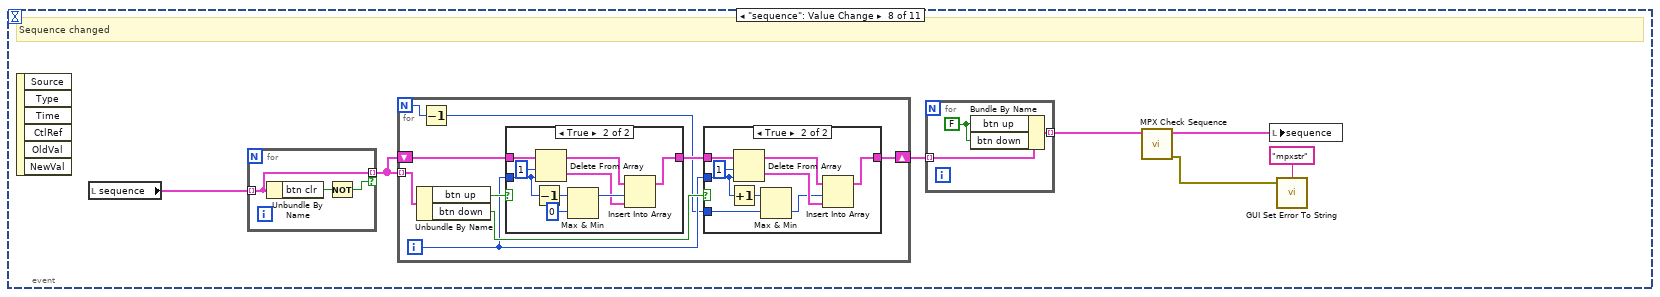
[diagram p13: hidden frame]
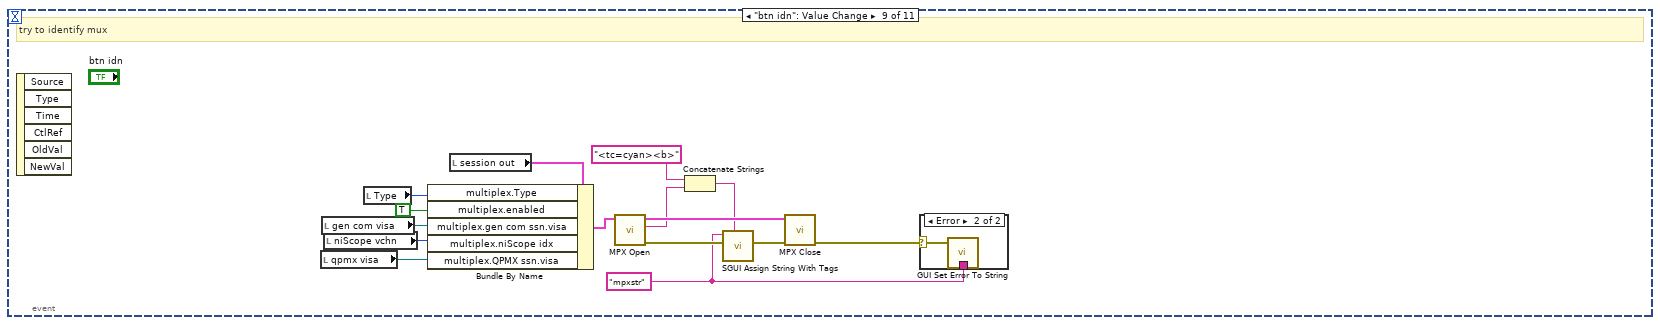
[diagram p16: hidden frame]
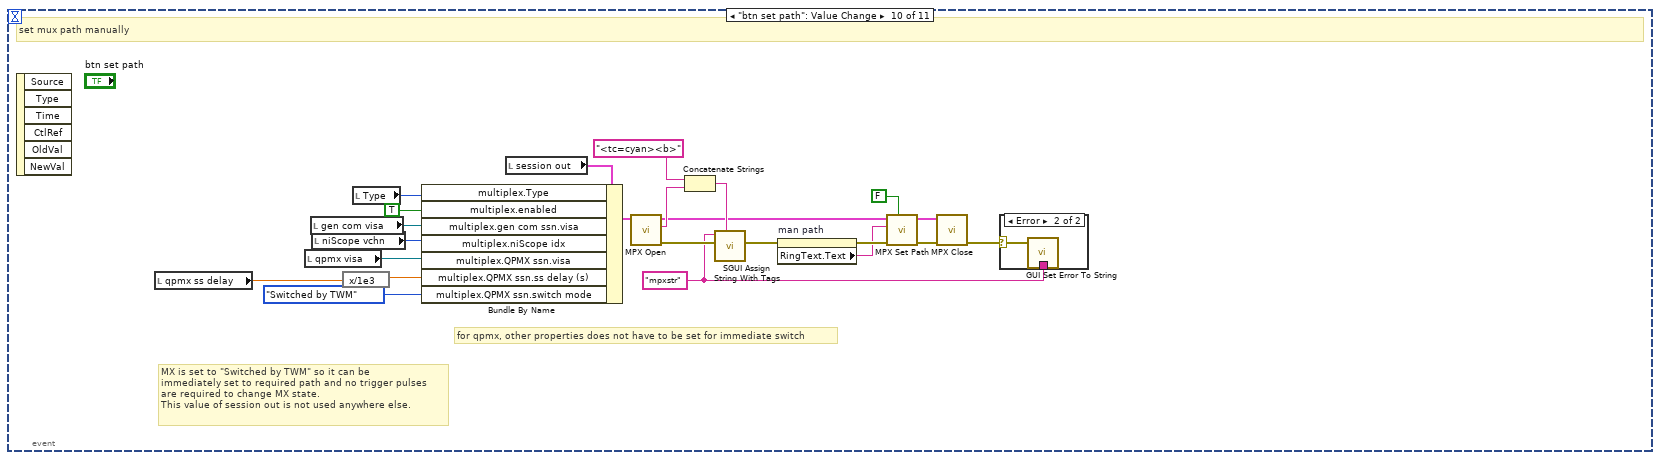
[diagram p18: hidden frame]
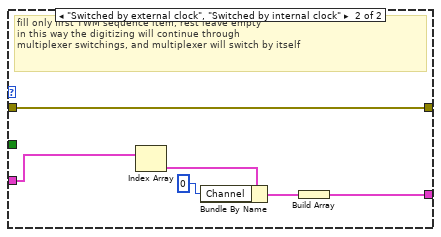
[diagram p20: hidden frame]
diagram:
  # "fill in sequence selector by last used"
  # "register controls on this panel\nfor GUI control, but don't\ndiscard main panel ones (add to stack)"
  n1 = call "align_vi_panel.vi"() -> ("error out"=w39:errorcluster)  [unwired: 11 in]
  n2 = call "SGUI Register Controls.vi"("error in"=w39, "register mode (overwrite)"=SGUI_Assign_References_Mode."Add to stack") -> ("assigned ID"=w37:string, "error out"=w35:errorcluster)  [unwired: 15 in, 1 out]
  n3 = Unbundle By Name("session in") -> ("multiplex.niScope idx"=w16:i32, "multiplex.Type"=w34:T60, "multiplex.gen com ssn"=w33:T61, "multiplex.delay before [s]"=w28:dbl, "multiplex.delay post [s]"=w27:dbl, "multiplex.sequence"=w22:string[], "multiplex.QPMX ssn"=w15:T65, "multiplex.VISA mux ssn"=w7:T68)
  n4 = call "MPX Get Path Names.vi"("session in"="session in") -> ("error out"=w25:errorcluster, "path tags"=w21:string[])  [unwired: 8 in, 1 out]
  n5 = control-ref of="sequence"() -> (w26:refnum<vi>)
  n6 = control-ref of="man path"() -> (w19:refnum<vi>)
  n7 = call "MPX Fill Sequence Selectors.vi"("manual path ref"=w19, "error in"=w25, "Strings []"=w21, "sequence ref"=w26) -> ("error out"=w18:errorcluster)  [unwired: 6 in, 1 out]
  n8 = local write "delay pre"(w28) -> ()
  n9 = local write "delay post"(w27) -> ()
  n10 = property on="Type" class="Enum (strict)"("Val(Sgnl)"=w34) -> ()  [unwired: 2 in, 2 out]
  n11 = call <vilib>:"Clear Errors.vi"("error in (no error)"=w18) -> ()  [unwired: 5 in, 2 out]
  n12 = Index Array(array="sequence") -> (element=w23:T81)  [unwired: 1 in]
  n13 = for {
    tunnel: w23 -> [w45]
    tunnel: w22 -> [w46] mode=indexing
    tunnel: w21 -> [w47]
    tunnel: [w42] -> w20 mode=indexing
    w43 = FALSE ("btn clr")
    n14 = Search 1D Array(1D array=w47, element=w46) -> (index of element=w44:i32)  [unwired: 1 in]
    n15 = Bundle By Name(cluster=w45, "btn clr"=w43, "btn up"=w43, "btn down"=w43, "Channel"=w44) -> (w42:T81)
  }
  n16 = Unbundle By Name(w33) -> ("visa"=w32:refnum<visa-resource-name>, "primary"=w31:T62, "secondary"=w30:T62, "channels"=w29:T63[])
  n17 = Unbundle By Name(w15) -> ("visa"=w14:refnum<visa-resource-name>, "switch mode"=w13:T66, "polarity"=w12:T67, "ss delay (s)"=w11:dbl, "internal timer (s)"=w9:dbl, "Last loaded sequence file"=w3:path, "timing delays"=w2:u32[])
  n18 = local write "error out"(w35) -> ()
  n19 = call <vilib>:"Clear Errors.vi"("error in (no error)"=w35) -> ("error out"=w38:errorcluster)  [unwired: 5 in, 1 out]
  n20 = while {
    tunnel: w38 -> [_]
    tunnel: [w48] -> w36
    stop <- w48 stop-if-true
    n21 = event shown="[10] \"qpmx load\", \"qpmx mode\": Value Change" {
      selector: _ -> [_ _ _ _ _ _ _ _ _ _ _]
      dyn-events: _ -> [_ _ _ _ _ _ _ _ _ _ _]
      timeout: _ -> [_ _ _ _ _ _ _ _ _ _ _]
      tunnel: [_ TRUE _ _ _ _ _ _ _ _ _] -> w48
      event Timeout {
        n22 = event-data() -> ()  [unwired: 1 in, 3 out]
      }
      event "btn ok", "btn cancel": Value Change; Panel Close {
        # "this one is just for debugging"
        n23 = event-data() -> ()  [unwired: 1 in, 3 out]
        n24 = local read "session out"() -> (w54:T1)
        n25 = local read "qpmx int timer"() -> (w57:i32)
        n26 = local read "qpmx ss delay"() -> (w58:dbl)
        n27 = Unbundle By Name(w54) -> ("multiplex.QPMX ssn"=w65:T65)
        n28 = Unbundle By Name(w54) -> ("multiplex.VISA mux ssn"=w53:T68)
        n29 = local read "qpmx polarity"() -> (w61:T67)
        n30 = To Double Precision Float(number=w57) -> (double precision float=w56:dbl)
        n31 = local read "qpmx mode"() -> (w60:T66)
        n32 = local read "com prim"() -> (w80:T62)
        n33 = local read "gen com visa"() -> (w81:refnum<visa-resource-name>)
        n34 = local read "com chan"() -> (w78:T63[])
        n35 = local read "com sec"() -> (w79:T62)
        n36 = local read "qpmx visa"() -> (w62:refnum<visa-resource-name>)
        n37 = expression code="x/1e3"(w56) -> (w55:dbl)
        n38 = expression code="x/1e3"(w58) -> (w59:dbl)
        n39 = local read "gen visa idn cmd"() -> (w49:string)
        n40 = local read "gen visa chans"() -> (w50:T69[])
        n41 = local read "gen visa visa"() -> (w51:refnum<visa-resource-name>)
        n42 = Unbundle By Name(w54) -> ("multiplex.gen com ssn"=w82:T61)
        n43 = Bundle By Name(cluster=w65, "visa"=w62, "switch mode"=w60, "polarity"=w61, "ss delay (s)"=w59, "internal timer (s)"=w55) -> (w63:T65)
        n44 = Bundle By Name(cluster=w82, "visa"=w81, "primary"=w80, "secondary"=w79, "channels"=w78) -> (w64:T61)
        n45 = Bundle By Name(cluster=w53, "VISA"=w51, "paths"=w50, "idn command"=w49) -> (w52:T68)
        n46 = local read "niScope vchn"() -> (w72:i32)
        n47 = local read "delay post"() -> (w76:dbl)
        n48 = local read "delay pre"() -> (w77:dbl)
        n49 = local read "Type"() -> (w83:T60)
        n50 = Bundle By Name(cluster=w54, "multiplex.Type"=w83, "multiplex.delay before [s]"=w77, "multiplex.delay post [s]"=w76, "multiplex.niScope idx"=w72, "multiplex.gen com ssn"=w64, "multiplex.QPMX ssn"=w63, "multiplex.VISA mux ssn"=w52) -> (w71:T1)
        n51 = local read "sequence"() -> (w75:T78)
        n52 = call "MPX Get Path Names.vi"("session in"=w71) -> ("error out"=w70:errorcluster, "path tags"=w69:string[], "session out"=w66:T1)  [unwired: 8 in]
        n53 = call <vilib>:"Clear Errors.vi"("error in (no error)"=w70) -> ()  [unwired: 5 in, 2 out]
        n54 = for {
          tunnel: w75 -> [w88] mode=indexing
          tunnel: [w86] -> w67 mode=indexing
          tunnel: w69 -> [w85]
          n55 = Unbundle By Name(w88) -> ("Channel"=w87:u16)
          n56 = Index Array(array=w85, index=w87) -> (element=w86:string)
        }
        n57 = Bundle By Name(cluster=w66, "multiplex.sequence"=w67) -> (w68:T1)
        n58 = Select(t=w68, s="btn ok", f=w54) -> (s? t:f=w73:T1)
        n59 = local write "session out"(w73) -> ()
        n60 = local write "session in"(w73) -> ()
      }
      event "tc device": Value Change {
        # "page select -> change type"
        n61 = event-data() -> ("NewVal"=w90:T79)  [unwired: 1 in, 5 out]
        n62 = local write "Type"(w90) -> ()
        n63 = local read "session out"() -> (w93:T1)
        n64 = local read "com chan"() -> (w100:T63[])
        n65 = property on="com chan" class="Arr"("Val(Sgnl)"=w100) -> (error out=w96:errorcluster)  [unwired: 2 in, 1 out]
        n66 = Bundle By Name(cluster=w93, "multiplex.Type"=w90) -> (w89:T1)
        n67 = call "MPX Get Path Names.vi"("error in"=w96, "session in"=w89) -> ("error out"=w95:errorcluster, "path tags"=w94:string[])  [unwired: 7 in, 1 out]
        n68 = control-ref of="sequence"() -> (w97:refnum<vi>)
        n69 = control-ref of="man path"() -> (w98:refnum<vi>)
        n70 = call "MPX Fill Sequence Selectors.vi"("manual path ref"=w98, "error in"=w95, "Strings []"=w94, "sequence ref"=w97) -> ("error out"=w92:errorcluster)  [unwired: 6 in, 1 out]
        n71 = local read "sequence"() -> (w99:T78)
        n72 = property on="sequence" class="Arr"(error in=w92, "Val(Sgnl)"=w99) -> (error out=w91:errorcluster)  [unwired: 1 in, 1 out]
        n73 = call <vilib>:"Clear Errors.vi"("error in (no error)"=w91) -> ()  [unwired: 5 in, 2 out]
      }
      event Value Change {
        # "Type changed"
        n74 = event-data() -> ("NewVal"=w101:T60)  [unwired: 1 in, 5 out]
        n75 = property on="tc device" class="TabCtl (strict)"("Val(Sgnl)"=w101) -> ()  [unwired: 2 in, 2 out]
      }
      event "btn gen visa cfg com": Value Change {
        # "setup COM port for generic VISA driver"
        n76 = event-data() -> ()  [unwired: 1 in, 6 out]
        n77 = local read "session out"() -> (w105:T1)
        n78 = Unbundle By Name(w105) -> ("multiplex.VISA mux ssn.serial cfg"=w106:T70)
        n79 = call "met_serial_cfg.vi"("dut serial in"=w106) -> ("error out"=w102:errorcluster, "dut serial out"=w104:T70)  [unwired: 9 in]
        n80 = Bundle By Name(cluster=w105, "multiplex.VISA mux ssn.serial cfg"=w104) -> (w103:T1)
        n81 = call <vilib>:"Clear Errors.vi"("error in (no error)"=w102) -> ()  [unwired: 5 in, 2 out]
        n82 = local write "session out"(w103) -> ()
      }
      event "gen visa chans": Value Change {
        # "change of VISA mux driver chnanels"
        n83 = event-data() -> ()  [unwired: 1 in, 6 out]
        n84 = local read "gen visa chans"() -> (w118:T69[])
        n85 = for {
          tunnel: w118 -> [w155] mode=indexing
          tunnel: [w155] -> w120 mode=indexing if=w153
          n86 = Unbundle By Name(w155) -> ("btn clr"=w154:bool)
          n87 = Not(x=w154) -> (.not. x?=w153:bool)
        }
        n88 = for {
          N -> [w126]
          tunnel: w120 -> [w131] mode=indexing
          shift-right: [w124] -> w119
          shift-left: w120 -> [w130]
          i -> [w127]
          n89 = Unbundle By Name(w131) -> ("btn up"=w132:bool, "btn down"=w128:bool)
          n90 = Decrement(x=w126) -> (x-1=w125:i32)
          n91 = case shown="True" w132 {
            tunnel: w130 -> [w143 w152]
            tunnel: w127 -> [_ w150]
            tunnel: [w143 w145] -> w129
            frame False {
            }
            frame True {
              n92 = Decrement(x=w150) -> (x-1=w144:i32)
              n93 = Delete From Array(array=w152, length=1, index=w150) -> (deleted portion=w146:T69[], array with subset deleted=w147:T69[])
              n94 = Max & Min(x=w144, y=0) -> (max(x,y)=w148:i32)  [unwired: 1 out]
              n95 = Insert Into Array(array=w147, index=w148, new element=w146) -> (w145:T69[])
            }
          }
          n96 = case shown="True" w128 {
            tunnel: w129 -> [w133 w142]
            tunnel: w127 -> [_ w140]
            tunnel: [w133 w137] -> w124
            tunnel: w125 -> [_ w136]
            frame False {
            }
            frame True {
              n97 = Increment(x=w140) -> (x+1=w134:i32)
              n98 = Delete From Array(array=w142, length=1, index=w140) -> (deleted portion=w138:T69[], array with subset deleted=w139:T69[])
              n99 = Max & Min(x=w134, y=w136) -> (min(x,y)=w135:i32)  [unwired: 1 out]
              n100 = Insert Into Array(array=w139, index=w135, new element=w138) -> (w137:T69[])
            }
          }
        }
        n101 = for {
          tunnel: w119 -> [w123] mode=indexing
          tunnel: [w121] -> w108 mode=indexing
          w122 = FALSE ("btn up")
          n102 = Bundle By Name(cluster=w123, "btn up"=w122, "btn down"=w122) -> (w121:T69)
        }
        n103 = local write "gen visa chans"(w108) -> ()
        n104 = local read "Type"() -> (w107:T60)
        n105 = local read "session out"() -> (w115:T1)
        n106 = Bundle By Name(cluster=w115, "multiplex.Type"=w107, "multiplex.VISA mux ssn.paths"=w108) -> (w114:T1)
        n107 = call "MPX Get Path Names.vi"("session in"=w114) -> ("error out"=w111:errorcluster, "path tags"=w112:string[], "session out"=w113:T1)  [unwired: 8 in]
        n108 = local write "session out"(w113) -> ()
        n109 = call <vilib>:"Clear Errors.vi"("error in (no error)"=w111) -> ("error out"=w110:errorcluster)  [unwired: 5 in, 1 out]
        n110 = control-ref of="sequence"() -> (w117:refnum<vi>)
        n111 = control-ref of="man path"() -> (w109:refnum<vi>)
        n112 = call "MPX Fill Sequence Selectors.vi"("manual path ref"=w109, "error in"=w110, "Strings []"=w112, "sequence ref"=w117) -> ("error out"=w116:errorcluster)  [unwired: 6 in, 1 out]
        n113 = call <vilib>:"Clear Errors.vi"("error in (no error)"=w116) -> ()  [unwired: 5 in, 2 out]
      }
      event "com chan": Value Change {
        w169 = "mpxstr" ("label(s) (status)")
        # "Generic COM - changed channel definitions"
        n114 = event-data() -> ()  [unwired: 1 in, 6 out]
        n115 = local read "com chan"() -> (w171:T63[])
        n116 = for {
          tunnel: w171 -> [w208] mode=indexing
          tunnel: [w208] -> w173 mode=indexing if=w206
          n117 = Unbundle By Name(w208) -> ("btn clr"=w207:bool)
          n118 = Not(x=w207) -> (.not. x?=w206:bool)
        }
        n119 = for {
          N -> [w179]
          tunnel: w173 -> [w184] mode=indexing
          shift-right: [w177] -> w172
          shift-left: w173 -> [w183]
          i -> [w180]
          n120 = Unbundle By Name(w184) -> ("btn up"=w185:bool, "btn down"=w181:bool)
          n121 = Decrement(x=w179) -> (x-1=w178:i32)
          n122 = case shown="True" w185 {
            tunnel: w183 -> [w196 w205]
            tunnel: w180 -> [_ w203]
            tunnel: [w196 w198] -> w182
            frame False {
            }
            frame True {
              n123 = Decrement(x=w203) -> (x-1=w197:i32)
              n124 = Delete From Array(array=w205, length=1, index=w203) -> (deleted portion=w199:T63[], array with subset deleted=w200:T63[])
              n125 = Max & Min(x=w197, y=0) -> (max(x,y)=w201:i32)  [unwired: 1 out]
              n126 = Insert Into Array(array=w200, index=w201, new element=w199) -> (w198:T63[])
            }
          }
          n127 = case shown="True" w181 {
            tunnel: w182 -> [w186 w195]
            tunnel: w180 -> [_ w193]
            tunnel: [w186 w190] -> w177
            tunnel: w178 -> [_ w189]
            frame False {
            }
            frame True {
              n128 = Increment(x=w193) -> (x+1=w187:i32)
              n129 = Delete From Array(array=w195, length=1, index=w193) -> (deleted portion=w191:T63[], array with subset deleted=w192:T63[])
              n130 = Max & Min(x=w187, y=w189) -> (min(x,y)=w188:i32)  [unwired: 1 out]
              n131 = Insert Into Array(array=w192, index=w188, new element=w191) -> (w190:T63[])
            }
          }
        }
        n132 = for {
          tunnel: w172 -> [w176] mode=indexing
          tunnel: [w174] -> w170 mode=indexing
          w175 = FALSE ("btn up")
          n133 = Bundle By Name(cluster=w176, "btn up"=w175, "btn down"=w175) -> (w174:T63)
        }
        n134 = local read "Type"() -> (w157:T60)
        n135 = call "GCOMM Check Channels"("channels in"=w170) -> ("error out"=w163:errorcluster, "channels out"=w164:T63[])  [unwired: 8 in, 1 out]
        n136 = local write "com chan"(w164) -> ()
        n137 = call-poly "SGUI Assign String With Tags.vi"("label(s) (empty)"="", "string (empty)"=w169) -> ()  [unwired: 8 in, 2 out]
        n138 = call "GUI Set Error To String.vi"("error in (no error)"=w163, "label(s) (status)"=w169) -> ()  [unwired: 3 in]
        n139 = local read "session out"() -> (w165:T1)
        n140 = Bundle By Name(cluster=w165, "multiplex.Type"=w157, "multiplex.gen com ssn.channels"=w164) -> (w162:T1)
        n141 = call "MPX Get Path Names.vi"("error in"=w163, "session in"=w162) -> ("error out"=w159:errorcluster, "path tags"=w160:string[], "session out"=w161:T1)  [unwired: 7 in]
        n142 = local write "session out"(w161) -> ()
        n143 = call <vilib>:"Clear Errors.vi"("error in (no error)"=w159) -> ("error out"=w158:errorcluster)  [unwired: 5 in, 1 out]
        n144 = control-ref of="sequence"() -> (w167:refnum<vi>)
        n145 = control-ref of="man path"() -> (w156:refnum<vi>)
        n146 = call "MPX Fill Sequence Selectors.vi"("manual path ref"=w156, "error in"=w158, "Strings []"=w160, "sequence ref"=w167) -> ("error out"=w166:errorcluster)  [unwired: 6 in, 1 out]
        n147 = call <vilib>:"Clear Errors.vi"("error in (no error)"=w166) -> ()  [unwired: 5 in, 2 out]
      }
      event "sequence": Value Change {
        # "Sequence changed"
        n148 = event-data() -> ()  [unwired: 1 in, 6 out]
        n149 = local read "sequence"() -> (w213:T78)
        n150 = for {
          tunnel: w213 -> [w250] mode=indexing
          tunnel: [w250] -> w215 mode=indexing if=w248
          n151 = Unbundle By Name(w250) -> ("btn clr"=w249:bool)
          n152 = Not(x=w249) -> (.not. x?=w248:bool)
        }
        n153 = for {
          N -> [w221]
          tunnel: w215 -> [w226] mode=indexing
          shift-right: [w219] -> w214
          shift-left: w215 -> [w225]
          i -> [w222]
          n154 = Unbundle By Name(w226) -> ("btn up"=w227:bool, "btn down"=w223:bool)
          n155 = Decrement(x=w221) -> (x-1=w220:i32)
          n156 = case shown="True" w227 {
            tunnel: w225 -> [w238 w247]
            tunnel: w222 -> [_ w245]
            tunnel: [w238 w240] -> w224
            frame False {
            }
            frame True {
              n157 = Decrement(x=w245) -> (x-1=w239:i32)
              n158 = Delete From Array(array=w247, length=1, index=w245) -> (deleted portion=w241:T78, array with subset deleted=w242:T78)
              n159 = Max & Min(x=w239, y=0) -> (max(x,y)=w243:i32)  [unwired: 1 out]
              n160 = Insert Into Array(array=w242, index=w243, new element=w241) -> (w240:T78)
            }
          }
          n161 = case shown="True" w223 {
            tunnel: w224 -> [w228 w237]
            tunnel: w222 -> [_ w235]
            tunnel: [w228 w232] -> w219
            tunnel: w220 -> [_ w231]
            frame False {
            }
            frame True {
              n162 = Increment(x=w235) -> (x+1=w229:i32)
              n163 = Delete From Array(array=w237, length=1, index=w235) -> (deleted portion=w233:T78, array with subset deleted=w234:T78)
              n164 = Max & Min(x=w229, y=w231) -> (min(x,y)=w230:i32)  [unwired: 1 out]
              n165 = Insert Into Array(array=w234, index=w230, new element=w233) -> (w232:T78)
            }
          }
        }
        n166 = for {
          tunnel: w214 -> [w218] mode=indexing
          tunnel: [w216] -> w212 mode=indexing
          w217 = FALSE ("btn up")
          n167 = Bundle By Name(cluster=w218, "btn up"=w217, "btn down"=w217) -> (w216:T81)
        }
        n168 = call "MPX Check Sequence.vi"("sequence in"=w212) -> ("error out"=w209:errorcluster, "sequence out"=w211:T78)  [unwired: 9 in]
        n169 = local write "sequence"(w211) -> ()
        n170 = call "GUI Set Error To String.vi"("error in (no error)"=w209, "label(s) (status)"="mpxstr") -> ()  [unwired: 3 in]
      }
      event "btn idn": Value Change {
        w255 = "mpxstr" ("label(s) (status)")
        # "try to identify mux"
        n171 = event-data() -> ()  [unwired: 1 in, 6 out]
        n172 = local read "qpmx visa"() -> (w251:refnum<visa-resource-name>)
        n173 = local read "gen com visa"() -> (w252:refnum<visa-resource-name>)
        n174 = local read "niScope vchn"() -> (w253:i32)
        n175 = local read "Type"() -> (w264:T60)
        n176 = local read "session out"() -> (w265:T1)
        n177 = Bundle By Name(cluster=w265, "multiplex.Type"=w264, "multiplex.enabled"=TRUE ("enabled"), "multiplex.gen com ssn.visa"=w252, "multiplex.niScope idx"=w253, "multiplex.QPMX ssn.visa"=w251) -> (w263:T1)
        n178 = call "MPX Open.vi"("session in"=w263) -> ("error out"=w258:errorcluster, "idn string"=w261:string, "session out"=w262:T1)  [unwired: 8 in]
        n179 = Concatenate Strings("<tc=cyan><b>" ("string"), w261) -> (w256:string)
        n180 = call-poly "SGUI Assign String With Tags.vi"("error in"=w258, "label(s) (empty)"=w255, "string (empty)"=w256) -> ("error out"=w257:errorcluster)  [unwired: 7 in, 1 out]
        n181 = call "MPX Close.vi"("error in"=w257, "session in"=w262) -> ("error out"=w259:errorcluster)  [unwired: 8 in, 1 out]
        n182 = case shown="Error" w259 {
          selector: w259 -> [_ w266]
          tunnel: w255 -> [_ w267]
          frame No Error {
          }
          frame Error {
            n183 = call "GUI Set Error To String.vi"("error in (no error)"=w266, "label(s) (status)"=w267) -> ()  [unwired: 3 in]
          }
        }
      }
      event "btn set path": Value Change {
        w283 = "mpxstr" ("label(s) (status)")
        # "for qpmx, other properties does not have to be set for immediate switch"
        # "MX is set to \"Switched by TWM\" so it can be\nimmediately set to required path and no trigger pulses\nare required to change MX state.\nThis value of session out is not used anywhere else."
        # "set mux path manually"
        n184 = event-data() -> ()  [unwired: 1 in, 6 out]
        n185 = local read "qpmx ss delay"() -> (w270:dbl)
        n186 = local read "qpmx visa"() -> (w271:refnum<visa-resource-name>)
        n187 = local read "gen com visa"() -> (w273:refnum<visa-resource-name>)
        n188 = local read "niScope vchn"() -> (w272:i32)
        n189 = expression code="x/1e3"(w270) -> (w269:dbl)
        n190 = local read "Type"() -> (w290:T60)
        n191 = local read "session out"() -> (w279:T1)
        n192 = Bundle By Name(cluster=w279, "multiplex.Type"=w290, "multiplex.enabled"=TRUE ("enabled"), "multiplex.gen com ssn.visa"=w273, "multiplex.niScope idx"=w272, "multiplex.QPMX ssn.visa"=w271, "multiplex.QPMX ssn.ss delay (s)"=w269, "multiplex.QPMX ssn.switch mode"=QPMX_switch_mode."Switched by TWM") -> (w289:T1)
        n193 = call "MPX Open.vi"("session in"=w289) -> ("error out"=w285:errorcluster, "idn string"=w288:string, "session out"=w278:T1)  [unwired: 8 in]
        n194 = Concatenate Strings("<tc=cyan><b>" ("string"), w288) -> (w284:string)
        n195 = call-poly "SGUI Assign String With Tags.vi"("error in"=w285, "label(s) (empty)"=w283, "string (empty)"=w284) -> ("error out"=w277:errorcluster)  [unwired: 7 in, 1 out]
        n196 = property on="man path" class="Ring (strict)"(error in=w277) -> (error out=w276:errorcluster, "RingText.Text"=w275:string)  [unwired: 1 in, 1 out]
        n197 = call "MPX Set Path.vi"("allow wait (True)"=FALSE, "error in"=w276, "path"=w275, "session in"=w278) -> ("error out"=w281:errorcluster, "session out"=w280:T1)  [unwired: 6 in]
        n198 = call "MPX Close.vi"("error in"=w281, "session in"=w280) -> ("error out"=w286:errorcluster)  [unwired: 8 in, 1 out]
        n199 = case shown="Error" w286 {
          selector: w286 -> [_ w291]
          tunnel: w283 -> [_ w292]
          frame No Error {
          }
          frame Error {
            n200 = call "GUI Set Error To String.vi"("error in (no error)"=w291, "label(s) (status)"=w292) -> ()  [unwired: 3 in]
          }
        }
      }
      event "qpmx load": Value Change {
        n201 = event-data() -> ("CtlRef"=w303:refnum<vi>)  [unwired: 1 in, 5 out]
        n202 = local read "session out"() -> (w312:T1)
        n203 = property class="Ctl"(reference=w303) -> ("ClassName"=w302:string)  [unwired: 1 in, 2 out]
        n204 = Equal?(x=w302, y="Boolean") -> (x = y?=w300:bool)
        n205 = case shown="True" w300 {
          tunnel: w312 -> [w330 w343]
          tunnel: [w330 w342] -> w297
          tunnel: [errorcluster {"status"=FALSE, "code"=0, "source"=""} ("error out") w331] -> w293
          frame False {
          }
          frame True {
            # "if error:\nImprove\nerror\nmessage"
            # "load sequences from file if button was pressed"
            n206 = call "Load Sequence from file.vi"("Sequence file path\n(file dialog if empty)"="qpmx file") -> ("error out"=w332:errorcluster, "Timing\ndelay"=w338:u32[], "Sequence"=w341:bool[][])  [unwired: 8 in]
            n207 = Unbundle By Name(w332) -> ("source"=w336:string)
            n208 = Format Into String(format string="Cannot load sequence file from path: \"%s\".\\n%s", "qpmx file", w336) -> (resulting string=w334:string)  [unwired: 2 in, 1 out]
            n209 = Bundle By Name(cluster=w343, "multiplex.QPMX ssn.sequence"=w341, "multiplex.QPMX ssn.timing delays"=w338, "multiplex.QPMX ssn.Last loaded sequence file"="qpmx file") -> (w342:T1)
            n210 = Bundle By Name(cluster=w332, "source"=w334) -> (w333:errorcluster)
            n211 = Array Size(array=w338) -> (size(s)=w340:i32)
            n212 = Select(t=w333, s=w332, f=w332) -> (s? t:f=w331:errorcluster)
            n213 = local write "qpmx loaded sequences"(w340) -> ()
            n214 = call "GUI Set Error To String.vi"("error in (no error)"=w331, "label(s) (status)"="mpxstr") -> ()  [unwired: 3 in]
          }
        }
        n215 = Bundle By Name(cluster=w297, "multiplex.QPMX ssn.switch mode"="qpmx mode") -> (w296:T1)
        n216 = Unbundle By Name(w296) -> ("multiplex.QPMX ssn.sequence"=w299:bool[][])
        n217 = call "MPX Get Path Names.vi"("error in"=w293, "session in"=w296) -> ("error out"=w308:errorcluster, "path tags"=w306:string[], "session out"=w307:T1)  [unwired: 7 in]
        n218 = local read "sequence"() -> (w295:T78)
        n219 = local write "session out"(w307) -> ()
        n220 = control-ref of="sequence"() -> (w310:refnum<vi>)
        n221 = control-ref of="man path"() -> (w311:refnum<vi>)
        n222 = call "MPX Fill Sequence Selectors.vi"("manual path ref"=w311, "error in"=w308, "Strings []"=w306, "sequence ref"=w310) -> ("error out"=w305:errorcluster)  [unwired: 6 in, 1 out]
        n223 = case shown="\"Switched by TWM\", Default" "qpmx mode" {
          tunnel: w305 -> [w319 w323]
          tunnel: [w319 w323] -> w304
          tunnel: [w318 w324] -> w294
          tunnel: w299 -> [w317 _]
          tunnel: w295 -> [w313 w328]
          frame "Switched by TWM", Default {
            # "fill out TWM sequences according the sequences in the file\nTWM will be switching the multiplexer"
            n224 = Array Size(array=w317) -> (size(s)=w315:i32[])
            n225 = Index Array(array=w313) -> (element=w316:T81)  [unwired: 1 in]
            n226 = Index Array(array=w315) -> (element=w314:i32)  [unwired: 1 in]
            n227 = for {
              N: w314 -> [_]
              tunnel: w316 -> [w322]
              tunnel: [w320] -> w318 mode=indexing
              i -> [w321]
              n228 = Bundle By Name(cluster=w322, "Channel"=w321) -> (w320:T81)
            }
          }
          frame "Switched by external clock", "Switched by internal clock" {
            # "fill only first TWM sequence item, rest leave empty\nin this way the digitizing will continue through\nmultiplexer switchings, and multiplexer will switch by itself"
            n229 = Index Array(array=w328) -> (element=w327:T81)  [unwired: 1 in]
            n230 = Bundle By Name(cluster=w327, "Channel"=u16 0) -> (w325:T81)
            n231 = Build Array(w325) -> (w324:T78)
          }
        }
        n232 = local write "sequence"(w294) -> ()
        n233 = property on="sequence" class="Arr"(error in=w304, "Val(Sgnl)"=w294) -> (error out=w309:errorcluster)  [unwired: 1 in, 1 out]
        n234 = call <vilib>:"Clear Errors.vi"("error in (no error)"=w309) -> ()  [unwired: 5 in, 2 out]
      }
    }
  }
  n235 = Unbundle By Name(w7) -> ("VISA"=w6:refnum<visa-resource-name>, "paths"=w5:T69[], "idn command"=w4:string)
  n236 = local write "niScope vchn"(w16) -> ()
  n237 = local write "com prim"(w31) -> ()
  n238 = local write "gen com visa"(w32) -> ()
  n239 = local write "com chan"(w29) -> ()
  n240 = local write "com sec"(w30) -> ()
  n241 = local write "sequence"(w20) -> ()
  n242 = local write "gen visa idn cmd"(w4) -> ()
  n243 = Array Size(array=w2) -> (size(s)=w1:i32)
  n244 = local write "gen visa chans"(w5) -> ()
  n245 = local write "gen visa visa"(w6) -> ()
  n246 = expression code="x*1e3"(w11) -> (w10:dbl)
  n247 = local write "qpmx visa"(w14) -> ()
  n248 = local write "qpmx mode"(w13) -> ()
  n249 = local write "qpmx polarity"(w12) -> ()
  n250 = expression code="x*1e3"(w9) -> (w8:dbl)
  n251 = local write "qpmx file"(w3) -> ()
  n252 = local write "qpmx loaded sequences"(w1) -> ()
  n253 = local write "qpmx ss delay"(w10) -> ()
  n254 = local write "qpmx int timer"(w8) -> ()
  n255 = flat-sequence {
    tunnel: w37 -> [w346]
    tunnel: w36 -> [_]
    frame #0 {
      # "on exit"
      n256 = call "SGUI Register Controls.vi"("register mode (overwrite)"=SGUI_Assign_References_Mode."Release ID", "controls ID (empty)"=w346) -> ("error out"=w345:errorcluster)  [unwired: 15 in, 2 out]
      n257 = call <vilib>:"Clear Errors.vi"("error in (no error)"=w345) -> ()  [unwired: 5 in, 2 out]
    }
  }
  "error out" <- "error in"
  "session out" <- "session in"
